vi "4ChNCS_BIOPAC_Zijing_amp_ph.vi"() -> ()   [LabVIEW 2016]
uses:
  <vilib>/measure/NI_MABase.lvlib
  <instrlib>/niUSRP/niUSRP Fetch Rx Data (2D CDB).vi
  <instrlib>/niUSRP/niUSRP Write Tx Data (2D CDB).vi
  <instrlib>/niUSRP/niUSRP Timestamp.ctl
  <instrlib>/niUSRP/niUSRP Configure Time Start Trigger.vi
  <vilib>/Analysis/NI_AALBase.lvlib
  <vilib>/Analysis/3filter.llb/Butterworth Filter (CDB).vi
  <vilib>/Analysis/3filter.llb/Filter Passband Type.ctl
  <vilib>/Analysis/3filter.llb/Butterworth Filter (DBL).vi
  C:/Program Files (x86)/BIOPAC Systems, Inc/BIOPAC Hardware API 2.2 Education/x64/mpdev.dll
  <vilib>/sound2/lvsound2.llb/Sampling Mode.ctl
  <vilib>/sound2/lvsound2.llb/Sound File Info (path).vi
  <vilib>/sound2/lvsound2.llb/Sound File Read Open.vi
  <vilib>/sound2/lvsound2.llb/Sound Output Write (DBL).vi
  <vilib>/sound2/lvsound2.llb/Sound File Read (DBL).vi
  <vilib>/Analysis/NI_AALPro.lvlib
  <vilib>/Platform/browser.llb/Open URL in Default Browser (string).vi
  <vilib>/Utility/miscctls.llb/LVDateTimeRec.ctl
panel:
  out "Wave size/ DS":dbl=10000.0 format="%#_6p"
  out "Tx ch1  ph":cdb[](array[numeric])
  out "Tx ch2  ph":cdb[](array[numeric])
  out "Tx ch4 ph":cdb[](array[numeric])
  out "Tx ch3  ph":cdb[](array[numeric])
  in  "Mute":bool
  out "Play Sound":bool=TRUE
  in  "bottom filter":T1
  in  "top filter":T1=enum."Bandpass"
  out "Acq Started":bool
  out "# BIO View Q":i32
  out "# BIO Buffer":i32
  out "Boolean":bool=TRUE
  out "Disconnecting":bool
  out "Stopping":bool
  out "Connecting":bool
  out "Disconnected":bool
  in  "Show BIO":bool
  out "# BIOViewQ2":i32
  out "Array 1 View":dbl[](graph)
  out "Array 2 View":dbl[](graph)
  out "Array 3 View":dbl[](graph)
  out "Array 4 View":dbl[](graph)
  out "View Array Size":i32
  out "# Elements in Array":i32
  out "ACQ -# Elements":i32
  out "Receive Success":bool
  out "# ACQ cycles":i32
  out "Bytes Read":i32
  out "Bytes To Read":i32
  out "Receive Total Size":dbl format="%#_13g"
  out "Receiving":bool
  in  "Start Acquisition":bool
  in  "Disconnect":bool
  out "ACQ ms":dbl=250.0 format="%#_13g"
  in  "Stop Acquisition":bool
  out "Connected":bool
  in  "Sample Rate":dbl=1.0 caption="ms/sample" min=0.0
  in  "Analog Channels":i32[](array[numeric])=[1, 1, 1, 1]
  out "# Channels":dbl format="%#_13g"
  out "BIO Connect":i32
  in  "BIO Connect":bool=TRUE
  in  "OpenHTML":bool=TRUE
  in  "Abd (cm)":string="0"
  in  "Thorax (cm)":string="0"
  in  "Comments":string
  in  "Weight (lbs)":string="0"
  in  "Age (yrs)":string="0"
  in  "Sex":string(combo)="Female"
  in  "Height (cm)":string="0"
  in  "Case #":string="14"
  out "Start Time":T2
  out "Total Routine Time":dbl(slide) scale=0.0..300.0
  out "Elapsed Time":dbl caption="Elapsed Time (s)"
  out "Next Instruction":string
  out "Current Instruction":string
  in  "Routine Selection":T3(ring)
  out "Current Routine":string
  out "Tx3Rx4":dbl[](graph)
  out "Tx4Rx3":dbl[](graph)
  out "ChAmp":dbl[][](array[numeric])=[[1.7262327066457893e-05, 1.899698926539768e-05, 2.131979680782845e-05, 2.7507513862708948e-05, 3.236234947998919e-05, 3.384280863448985e-05, 3.3113712649913256e-05, 2.8744318806479064e-05, 2.4117959107532184e-05, 2.0714217164135817e-05, 1.7964639969242282e-05, 1.4127881869429752e-05, 1.5692535768228094e-05, 2.4152619914305532e-05, 2.8339686382715385e-05, 2.606906286720416e-05, 2.1755918570529384e-05, 2.0929028564145826e-05, 2.2419410493859248e-05, 2.1786896096171967e-05, 1.7145005999174206e-05, 1.5886785364638103e-05, 1.995380091360238e-05, 1.96084446445408e-05, 1.3881312052638574e-05, 5.368463432831762e-06, 7.886976522489036e-06, 1.718108126568357e-05, 1.984430714817916e-05, 1.8874058751572535e-05, 1.7869312672433515e-05, 1.7356735499504872e-05, 2.065235332503479e-05, 2.1951680154988656e-05, 2.0363547237431346e-05, 2.1229264430323524e-05, 2.188656276617781e-05, 2.1477411495382004e-05, 1.913194947952161e-05, 1.374906879007994e-05, 1.084407557924396e-05, 1.0538448835067238e-05, 1.3462486513328936e-05, 1.979383250422823e-05, 2.381539261154395e-05, 2.2167223174073578e-05, 1.7644503717147575e-05, 1.870536234643517e-05, 2.2751950524913166e-05, 2.340432192813861e-05, 2.2468849270761083e-05, 2.4188550691353842e-05, 2.7519058552290856e-05, 3.1102581077866726e-05, 3.580393911829494e-05, 3.78912649503874e-05, 3.327873597801261e-05, 2.4510981949940783e-05, 1.8465065354817837e-05, 1.7132224969133005e-05, 1.7642310138371268e-05, 1.88142956741822e-05, 1.560032046277488e-05, 9.753217862235494e-06, 1.2015090850038981e-05, 1.776834560720681e-05, 2.4803861691952522e-05, 2.8043624192078222e-05, 2.684382525540612e-05, 2.3530222840588965e-05, 2.0528849124310057e-05, 1.9668374613316667e-05, 1.9146637114645684e-05, 1.5474488036915515e-05, 1.739488550213199e-05, 2.5095299380068926e-05, 3.2858145215540916e-05, 3.439509649081835e-05, 2.6143868318774837e-05, 1.7977385637690134e-05, 1.6384181575586158e-05, 1.4888284293264162e-05, 1.1597491470576354e-05, 1.1445555578759772e-05, 1.4980688444081562e-05, 1.909173519498907e-05, 1.9461150455264684e-05, 1.845876729070065e-05, 1.8005010185132642e-05, 1.9028924898462435e-05, 1.7575955788217445e-05, 1.4184298105937452e-05, 9.414371560237339e-06, 5.4356042784590255e-06, 8.10928562517548e-06, 9.28876849225871e-06, 8.695785214389758e-06, 1.2695777397634576e-05, 1.6809431598631123e-05, 2.1908643727461497e-05], [0.39904903865563796, 0.39903176051530775, 0.39902405260596024, 0.3990221650023599, 0.3990182934858042, 0.39901299641778676, 0.39900459263010085, 0.39899398548309095, 0.3989851312683333, 0.3989817758172843, 0.39898441600096285, 0.3989920701551657, 0.3989957319087615, 0.3989970252526829, 0.3990014639144786, 0.3990082495650084, 0.39901677157837184, 0.39902202434845035, 0.3990170521098724, 0.3990061914814684, 0.39899957115083645, 0.39900163440594105, 0.39901134932465093, 0.3990245430143365, 0.3990299364956871, 0.3990206423396574, 0.39901294696264844, 0.399015237964853, 0.3990195320664335, 0.3990239908891069, 0.39902678858482366, 0.3990303142377581, 0.3990363654196349, 0.39903798034344395, 0.39903568308022536, 0.3990295778239386, 0.3990213145612541, 0.3990115641317417, 0.3990031911721688, 0.3990044335692754, 0.3990142055365442, 0.3990231880559529, 0.3990294810791408, 0.39903152543597487, 0.3990303417237137, 0.39902587131491124, 0.39902317862698444, 0.3990231908517323, 0.3990187535042287, 0.39901147460102687, 0.39900466569609977, 0.399000198693456, 0.398994572076958, 0.39898792975360287, 0.39898351183081265, 0.39898252129559103, 0.3989860199605185, 0.3989908704807006, 0.39899345184972185, 0.39899268675930705, 0.39898929894357515, 0.39898974479144206, 0.3989970434213525, 0.39900457970685, 0.3990084272376425, 0.3990059437407563, 0.39900092658003017, 0.3989998521554356, 0.3989999155043143, 0.39900335732390085, 0.3990086633280822, 0.39901161043288735, 0.3990153435576799, 0.3990232290578827, 0.39902895125044885, 0.3990233171970213, 0.39901091768095076, 0.3989963560226853, 0.3989823146041765, 0.39898013105698543, 0.39899131681473166, 0.3990088743561722, 0.39902163871137375, 0.39902552269435965, 0.3990216751013488, 0.3990108271690995, 0.3989999368161602, 0.39899179748001445, 0.3989869444795569, 0.3989823014007489, 0.3989811018380635, 0.3989866085692465, 0.3989974881575293, 0.399009653455826, 0.39902039237597164, 0.39903113834388676, 0.39903799466445666, 0.39903656085835637, 0.39902912933239515, 0.3990196685727854], [0.5089284260094796, 0.5089413529092005, 0.5089385924023097, 0.5089461735853302, 0.5089333321440155, 0.5089367652503622, 0.5089376331435306, 0.5089306671430541, 0.508949239645895, 0.5089486561361645, 0.5089529378833244, 0.5089419476875585, 0.5089298840108731, 0.5089475772042052, 0.5089441426339854, 0.5089427381450184, 0.5089483329108746, 0.5089280151098653, 0.5089336602793385, 0.5089062019851882, 0.5089074628030626, 0.5088932174425751, 0.5088701289561509, 0.5088760830698362, 0.5088683341509143, 0.5088818393635381, 0.5089000365985035, 0.5088962730652971, 0.5089053012825656, 0.5088919060061875, 0.5088858810710211, 0.5088778714303226, 0.508862396898039, 0.5088799706522465, 0.508890020250467, 0.5089068411749241, 0.508910151200762, 0.5088879724716624, 0.5088963605339264, 0.5088989546591678, 0.5089079531975655, 0.5089307483176185, 0.5089353690581762, 0.5089322510910641, 0.5089226818391756, 0.5089231205950179, 0.5089421889187917, 0.5089302121637822, 0.5089288553338916, 0.5089136387417116, 0.5088923938634197, 0.5088806790242092, 0.5088543127997475, 0.5088388632427274, 0.5088290815518671, 0.5088136498514574, 0.508828716232115, 0.5088373004254244, 0.5088536031198835, 0.5088663652543981, 0.5088663647379902, 0.5088663839922184, 0.5088589552438861, 0.5088642449634635, 0.5088725023266256, 0.5088718014416865, 0.5088674063260687, 0.5088515437004615, 0.5088682831786894, 0.5088713788197812, 0.5088809924897628, 0.508878513506942, 0.5088771181893693, 0.5088848435184512, 0.5088770842370816, 0.5088914766511436, 0.5089003523667647, 0.5089066301516674, 0.5089314320882471, 0.5089402101447223, 0.508962553406896, 0.5089753861787446, 0.5089593307295952, 0.5089478542324088, 0.5089278310589712, 0.5089248500720587, 0.5089163513653545, 0.5089005689237424, 0.5089083211616405, 0.5088993300683022, 0.5088927412237987, 0.5088830866377116, 0.5088718481995638, 0.5088897909905771, 0.5088809733102648, 0.5088790935282286, 0.5088680814653207, 0.5088523600270333, 0.5088613943195607, 0.5088543176402154], [2.0662941946213977e-05, 2.282608405319783e-05, 2.237600508813514e-05, 2.2542693256186783e-05, 2.041826329305299e-05, 1.6288400811782785e-05, 1.0891495139698275e-05, 1.4190599881567273e-05, 1.8742691366266016e-05, 1.8736119036749436e-05, 1.741774537028846e-05, 1.5658954058158222e-05, 1.5904856683822096e-05, 1.6871005066910787e-05, 1.5599249074465836e-05, 1.3520520470394872e-05, 1.3927163947888679e-05, 1.5334805249818678e-05, 1.4564830067379515e-05, 9.817520346860189e-06, 1.3098820613974226e-05, 1.929550220456421e-05, 2.3072255815616586e-05, 2.4321951176986116e-05, 2.3250917563816834e-05, 2.1644284217119052e-05, 1.7041306350033735e-05, 1.0688883027066213e-05, 9.28433634468159e-06, 1.1420718289762068e-05, 1.7056250213804775e-05, 1.9836991189555113e-05, 1.746716828521344e-05, 1.2441527630540996e-05, 8.566795426917848e-06, 9.815076354382859e-06, 1.0229272880058857e-05, 9.936691802926115e-06, 1.536494187514889e-05, 2.3346259934086635e-05, 2.7477587888222747e-05, 2.882421007601368e-05, 2.763067836551142e-05, 2.1577345489474273e-05, 1.3485424327083916e-05, 9.52579824483287e-06, 1.3113651673496717e-05, 1.5276095683726537e-05, 1.6308973250379756e-05, 1.8045078515596545e-05, 1.7849042225306495e-05, 1.2607829522468473e-05, 7.109107971268437e-06, 6.6038815895810515e-06, 6.924972052119899e-06, 4.965235247536195e-06, 5.757305113334596e-06, 9.21497446069365e-06, 9.781248515919794e-06, 1.0683021318304504e-05, 1.196938592791573e-05, 1.159802409297526e-05, 1.012272777630437e-05, 9.65935822948268e-06, 1.4116839432017005e-05, 1.847684147148342e-05, 1.6783927528588872e-05, 1.0863513026975652e-05, 7.650914818223192e-06, 9.456183557358687e-06, 1.0426180609097815e-05, 8.567604650724215e-06, 8.546559610017728e-06, 1.2946532793024891e-05, 1.7245567743458815e-05, 2.0097444147186203e-05, 2.0459407417437442e-05, 1.9957232554286306e-05, 1.996659645997603e-05, 1.7332136966233293e-05, 1.5115608112097958e-05, 1.762095864401886e-05, 1.992020410454883e-05, 2.0585166404108466e-05, 2.212056735942569e-05, 2.2957279986002272e-05, 2.3103396847026532e-05, 2.320807116373638e-05, 2.0818984342366494e-05, 1.789850158592137e-05, 1.64936985167028e-05, 1.4204813599995013e-05, 1.2878752736428332e-05, 1.4757379916553103e-05, 1.713867099725903e-05, 1.6105166890214558e-05, 1.20593443919334e-05, 1.2171370167939264e-05, 1.2336933066341984e-05, 1.1620987924410626e-05]]
  out "Output":bool=TRUE
  out "Ch4 Amplitude":dbl step=0.05 format="%#.6g"
  out "Ch3 Amplitude":dbl=0.25 step=0.05 format="%#.6g"
  out "Ch2 Amplitude":dbl=0.6 step=0.05 format="%#.6g"
  out "Ch1 Amplitude":dbl step=0.05 format="%#.6g"
  out "Tx1Rx2":dbl[](graph)
  out "Tx2Rx1":dbl[](graph)
  out "Dis Sampling Rate":dbl=1000.0 format="%#_6p"
  in  "DownSamplingRatio 2":i32=10
  out "Sampling Rate":dbl=10000.0 format="%#_6p"
  out "Flush":bool
  out "8 Ch Heart":dbl[][](array[numeric])
  out "NCS Save Loops":i32=56132
  out "Save":bool
  out "# NCS Buffer":i32
  out "Buffer":bool
  in  "fl Bottom":dbl=10.0 format="%0.4f"
  in  "fh Bottom":dbl=20.0 format="%0.2f"
  in  "DownSamplingRatio1":i32=200
  in  "fl Top":dbl=4.0 format="%0.4f"
  in  "fh Top":dbl=20.0 format="%0.2f"
  out "# elements in view queue":i32
  out "DownSamplingRatio":i32=100
  out "BW/2":dbl=1000.0
  out "# IQ queue Ch 2":i32
  out "# IQ queue Ch 1":i32
  in  "Dis2":bool=TRUE
  in  "Dis1":bool=TRUE
  out "IQ Graph 2":dbl[][](graph)
  out "IQ Graph":dbl[][](graph)
  out "Tx2 Waveform":cdb[][](array[numeric])
  out "Tx1 Waveform":cdb[][](array[numeric])
  in  "Ch3&4 carrier frequency [Hz] 2":dbl=1000000000.0 format="%#_6p"
  in  "Ch1&2 carrier frequency [Hz]":dbl=900000000.0 format="%#_6p"
  in  "Rx2 Gain 2":dbl=15.0 format="%#_6f"
  in  "Tx2 Gain 2":dbl=20.0 format="%#_6f"
  in  "Rx1 Gain 2":dbl=15.0 format="%#_6f"
  in  "Tx1 Gain 2":dbl=20.0 format="%#_6f"
  out "error out 2":errorcluster
  in  "Start Trigger Time 2":T4={"whole seconds"=1, "fractional seconds"=0.0}
  in  "Channel 4 Tone Amplitude":dbl=0.5 step=0.05 format="%#.6g"
  in  "Channel 4 Tone Frequency":dbl=430000.0 format="%#_6p"
  in  "Channel 3 Tone Amplitude":dbl=0.5 step=0.05 format="%#.6g"
  in  "Channel 3 Tone Frequency":dbl=473000.0 format="%#_6p"
  out "Tx2 Waveform Graph":waveform(dbl)[](graph)=[{"t0"=timestamp(0.45999999999999996 s since 1904-01-01), "dt"=1e-06, "Y"=array[10000 elements]}, {"t0"=timestamp(0.45999999999999996 s since 1904-01-01), "dt"=1e-06, "Y"=array[10000 elements]}, {"t0"=timestamp(0.45999999999999996 s since 1904-01-01), "dt"=1e-06, "Y"=array[10000 elements]}, {"t0"=timestamp(0.45999999999999996 s since 1904-01-01), "dt"=1e-06, "Y"=array[10000 elements]}]
  in  "Waveform Size 2":dbl=10000.0
  in  "Stop 2":bool
  in  "Device Name 2":refnum<k15>="MyB210_2"
  in  "Tx2 Gain 1":dbl=20.0 format="%#_6f"
  in  "Tx IQ Rate 2":dbl=1000000.0 format="%#_6p"
  in  "Rx2 Gain 1":dbl=15.0 format="%#_6f"
  in  "Rx IQ Rate 2":dbl=1000000.0 format="%#_6p"
  out "error out 1":errorcluster
  in  "Start Trigger Time":T4={"whole seconds"=1, "fractional seconds"=0.0}
  in  "Stop":bool
  in  "Channel 2 Tone Amplitude":dbl=0.5 step=0.05 format="%#.6g"
  in  "Channel 2 Tone Frequency":dbl=440000.0 format="%#_6p"
  in  "Channel 1 Tone Amplitude":dbl=0.5 step=0.05 format="%#.6g"
  in  "Channel 1 Tone Frequency":dbl=355000.0 format="%#_6p"
  out "Tx1 Waveform Graph":waveform(dbl)[](graph)=[{"t0"=timestamp(0.45999999999999996 s since 1904-01-01), "dt"=1e-06, "Y"=array[10000 elements]}, {"t0"=timestamp(0.45999999999999996 s since 1904-01-01), "dt"=1e-06, "Y"=array[10000 elements]}, {"t0"=timestamp(0.45999999999999996 s since 1904-01-01), "dt"=1e-06, "Y"=array[10000 elements]}, {"t0"=timestamp(0.45999999999999996 s since 1904-01-01), "dt"=1e-06, "Y"=array[10000 elements]}]
  in  "Waveform Size 1":dbl=10000.0
  in  "Device Name":refnum<k15>="MyB210_1"
  in  "Tx1 Gain 1":dbl=20.0 format="%#_6f"
  in  "Tx IQ Rate 1":dbl=1000000.0 format="%#_6p"
  in  "Rx1 Gain 1":dbl=15.0 format="%#_6f"
  in  "Rx IQ Rate 1":dbl=1000000.0 format="%#_6p"
  # "Misc"
  # "Tx Waveform"
  # "IQ waveform"
  # "NCS"
  # "Channel Settings"
  # "Channel 1"
  # "Device Settings"
  # "BIO"
  # "Channel 2"
  # "Filters"
  # "Buffers"
  # "BIOPAC Connection"
  # "Channel 3"
  # "Post Study Survey:"
  # "https://cornell.qualtrics.com/jfe/form/SV_9QryoqkUKquSXD7"
  # "Channel 4"
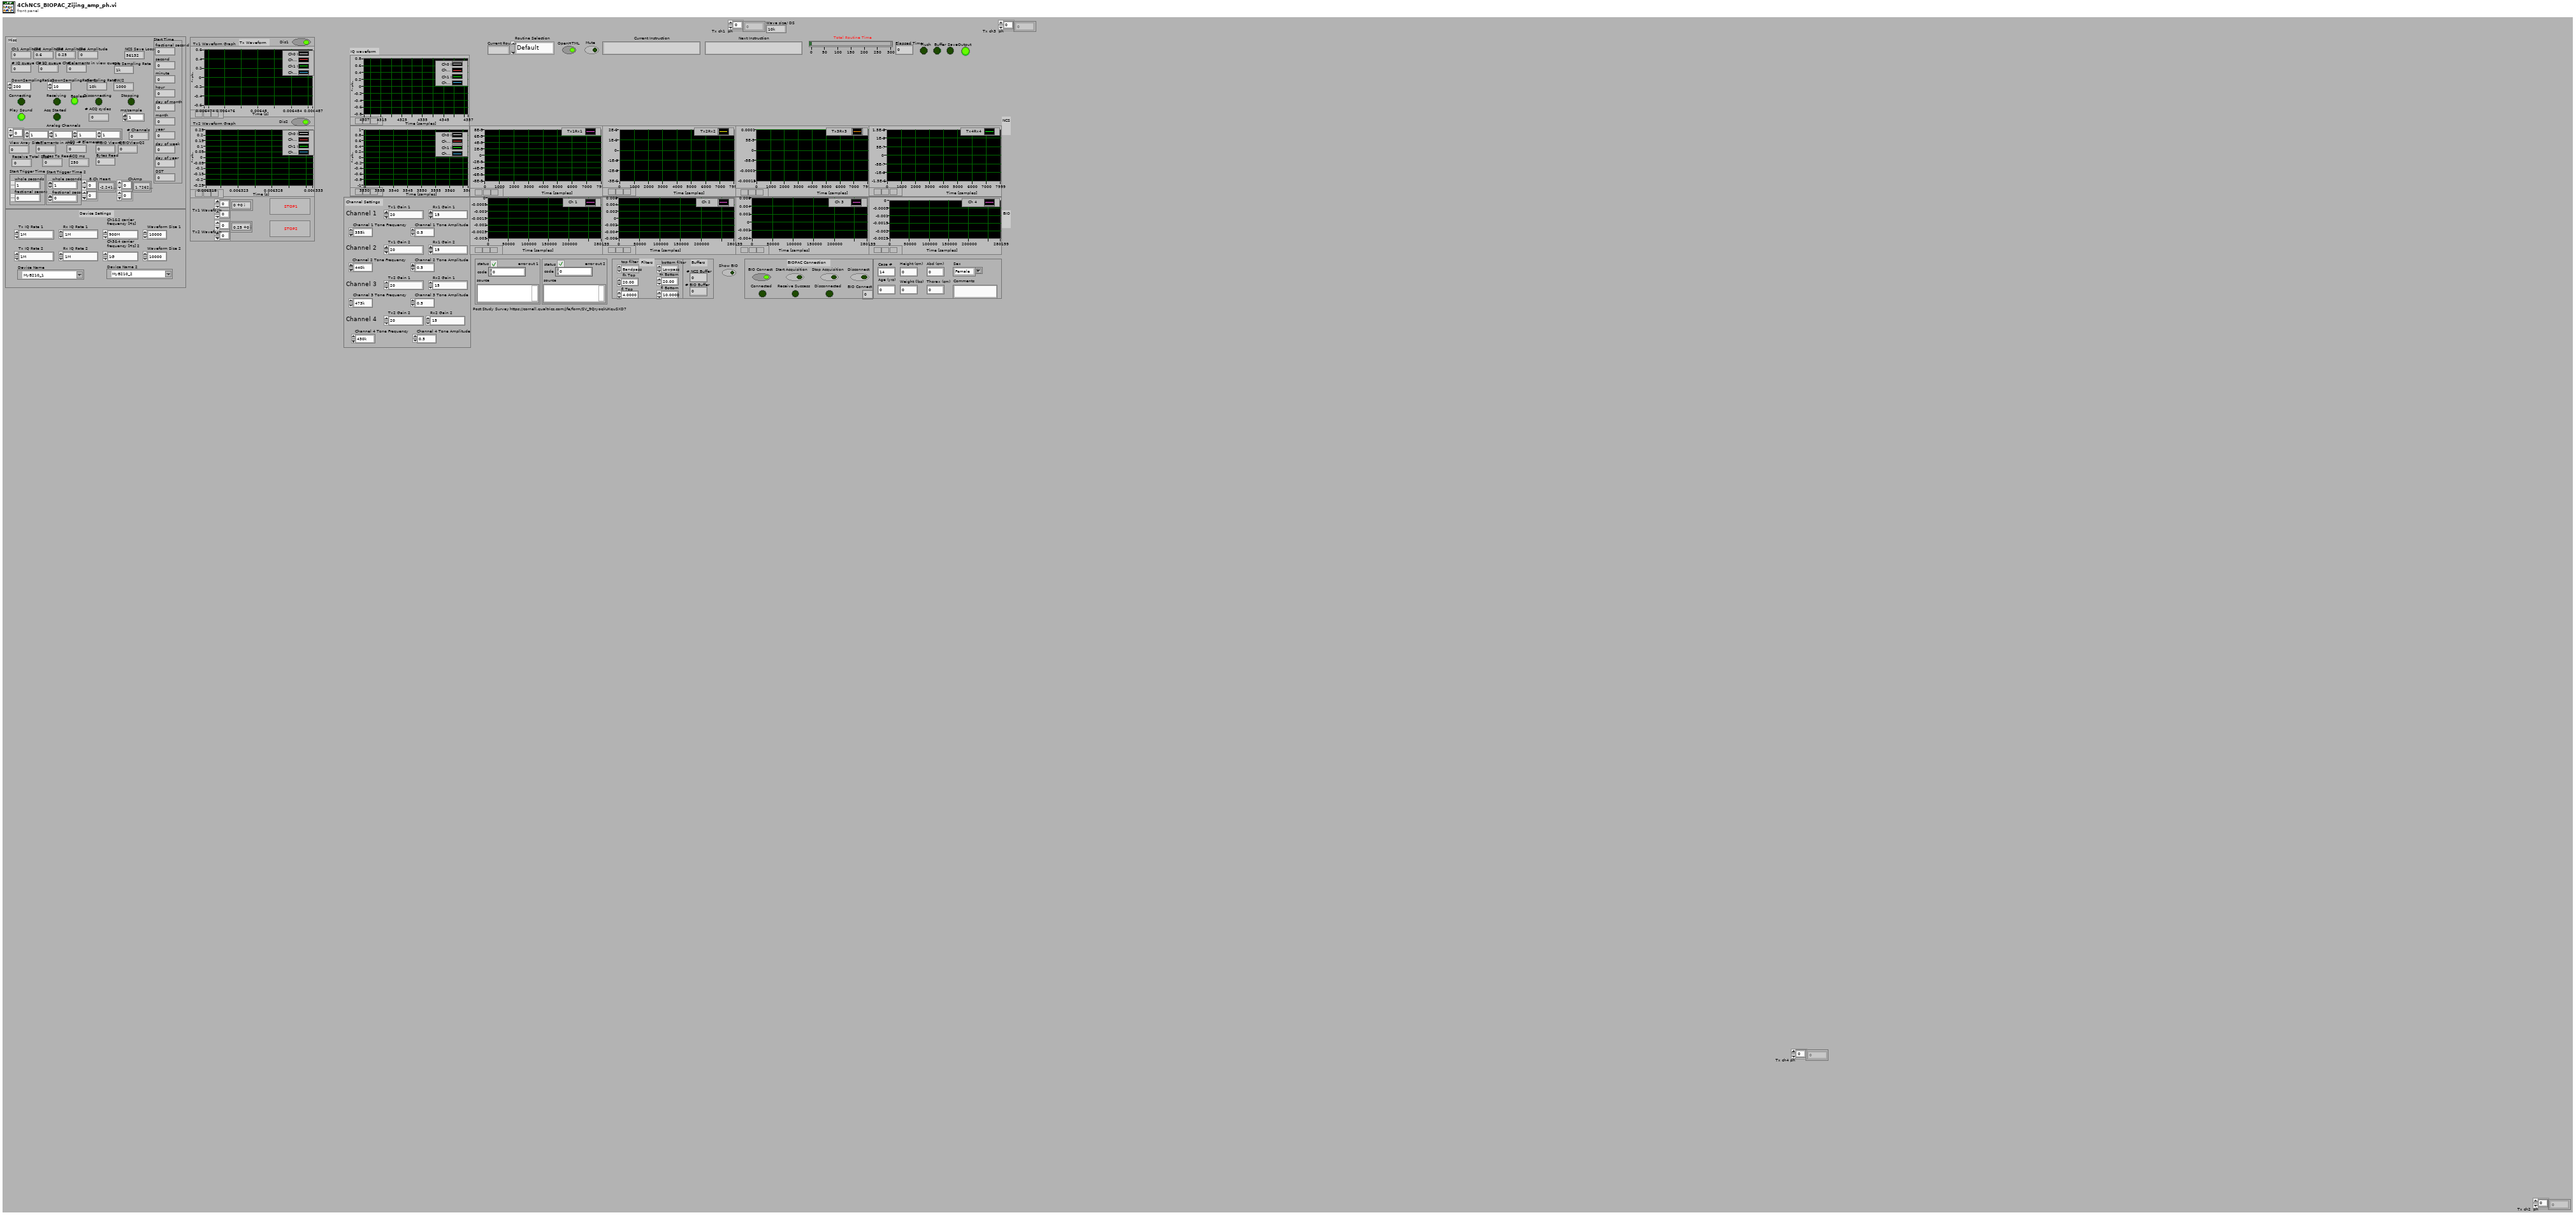
[diagram p1: front panel]
types:
  T1 = typedef "NI_AALBase.lvlib/Filter Passband Type.ctl" = enum32{"Lowpass", "Highpass", "Bandpass", "Bandstop"}
  T2 = typedef "LVDateTimeRec.ctl" = cluster{"fractional second":dbl, "second":i32, "minute":i32, "hour":i32, "day of month":i32, "month":i32, "year":i32, "day of week":i32, "day of year":i32, "DST":i32}
  T3 = enum16{"Default", "Test Run", "Training", "Routine 1", "Routine 2", "Routine 3", "Routine 4", "Routine 5a", "Routine 5b"}
  T4 = typedef "niUSRP Timestamp.ctl" = cluster{"whole seconds":u64, "fractional seconds":dbl}
  T5 = typedef "Sampling Mode.ctl" = i32
  T6 = typedef "Sound Data Format.ctl" = cluster{"sample rate (S/s)":dbl, "number of channels":i32, "bits per sample":i32}
  T7 = typedef "Sound File Refnum.ctl" = refnum<file>
  T8 = typedef "Sound Output Task ID.ctl" = u32
  T9 = enum16{"open", "open or create", "create or replace", "create", "open (read-only)"}
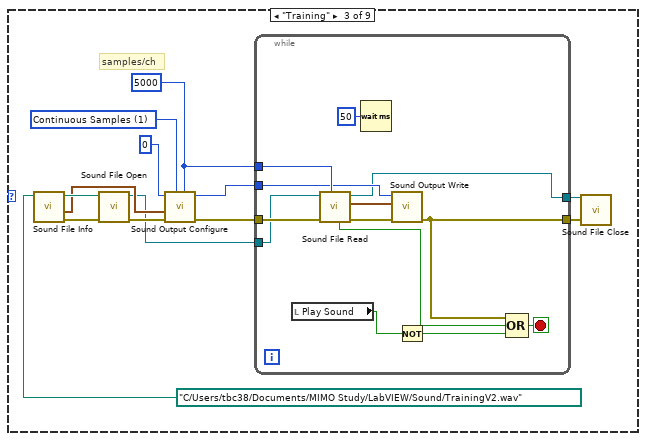
[diagram p4: hidden frame]
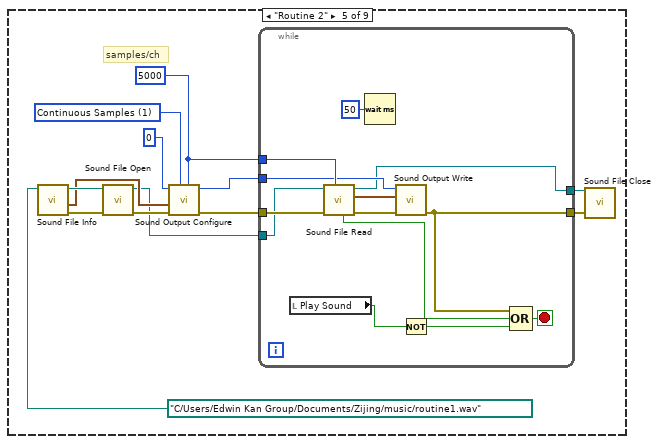
[diagram p6: hidden frame]
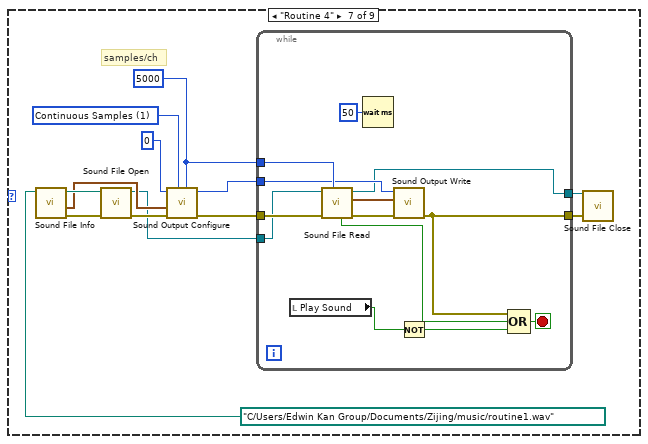
[diagram p8: hidden frame]
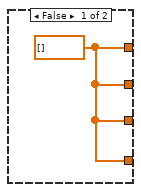
[diagram p11: hidden frame]
diagram:
  w1 = FALSE
  w29 = enum16{"Default"}."Default"
  w26 = 0.0 ("element")
  w27 = 800 ("dimension size")
  w33 = 4 ("dimension size")
  (unwired) 10
  w85 = "RX2"  # Tx active antenna
  w86 = "RX2"  # Tx active antenna
  w142 = 1 items=["Now", "Next Timebase Edge"] ("apply timestamp")
  w114 = "TX1"  # Tx active antenna
  w208 = 1 items=["Now", "Next Timebase Edge"] ("apply timestamp")
  w180 = "TX1"  # Tx active antenna
  # "Sound"
  # "Get it so that it acquires the proper number of cycles for the routine time. Front should be save synchronized"
  # "BIOPAC QUEUE"
  # "Current Sync Method:\nStart Buffering as soon as Acquisition Starts"
  # "Biopac Code. Use the flags to switch between these loops.\nCONNECT- Run to connect to the BIOPAC. Acquisition will not start. 'Connect Success' returns the status of this function.\nSTART ACQUISITION- Run to begin acquiring data from the BIOPAC. SYNCHRONIZATION IS IMPORTANT HERE.\nSTOP ACQUISITION- Run to stop acquiring data. The BIOPAC will disconnect and reconnect to prepare for another acquisition.\nDISCONNECT- Run to disconnect from BIOPAC. This will prohibit connection until the VI is restarted.\nSHOW/VIEWING- Dequeues the elements and displays them."
  # "Routine selection and implementation Loop"
  # "DownSamplingRatio"
  # "Set the attributes \nspecific to channel 1."
  # "Set the attributes \nspecific to channel 0."
  # "Set the attributes \nused by both Rx channels"
  # "Set the attributes \nspecific to Rx channel 1."
  # "Set the attributes \nspecific to Rx channel 0."
  # "Set the attributes \nspecific to channel 1."
  # "Set the attributes \nspecific to channel 0."
  # "Set the attributes \nused by both Rx channels"
  # "Set the attributes \nspecific to Rx channel 1."
  # "Set the attributes \nspecific to Rx channel 0."
  n1 = local write "BIO Connect"(w1) -> ()
  n2 = local write "Start Acquisition"(w1) -> ()
  n3 = local write "Stop Acquisition"(w1) -> ()
  n4 = local write "Disconnect"(w1) -> ()
  n5 = local write "Show BIO"(w1) -> ()
  n6 = local read "Device Name 2"() -> (w150:refnum<k15>)
  n7 = while {
    stop <- FALSE stop-if-true
    n8 = Wait (ms)(milliseconds to wait=50) -> ()  [unwired: 1 out]
    n9 = Not(x="Mute") -> (.not. x?=w224:bool)
    n10 = case shown="True" w224 {
      frame False {
      }
      frame True {
        n11 = local read "Routine Selection"() -> (w227:T3)
        n12 = case shown="\"Default\", Default" w227 {
          frame "Default", Default {
          }
          frame "Test Run" {
          }
          frame "Training" {
            w231 = 5000
            w234 = T5 1 items=["Finite Samples", "Continuous Samples"] ("sample mode")
            # "samples/ch"
            n13 = call-poly <vilib>:"Sound File Info.vi"("path"=path "C:/Users/tbc38/Documents/MIMO Study/LabVIEW/Sound/TrainingV2.wav") -> ("error out"=w239:errorcluster, "sound format"=w235:T6, "path out"=w240:path)  [unwired: 7 in, 1 out]
            n14 = call-poly <vilib>:"Sound File Open.vi"("error in (no error)"=w239, "path"=w240) -> ("error out"=w238:errorcluster, "sound file refnum"=w230:T7)  [unwired: 8 in]
            n15 = call <vilib>:"Sound Output Configure.vi"("number of samples/ch"=w231, "sample mode"=w234, "error in (no error)"=w238, "sound format"=w235, "device ID"=u32 0) -> ("error out"=w233:errorcluster, "task ID"=w232:T8)  [unwired: 5 in]
            n16 = while {
              tunnel: w233 -> [w251]
              tunnel: w232 -> [w252]
              tunnel: w231 -> [w253]
              tunnel: w230 -> [w250]
              tunnel: [w244] -> w229
              tunnel: [w248] -> w228
              stop <- w242 stop-if-true
              n17 = local read "Play Sound"() -> (w241:bool)
              n18 = call-poly <vilib>:"Sound File Read.vi"("number of samples/ch (-1: all)"=w253, "error in (no error)"=w251, "sound file refnum"=w250) -> ("error out"=w247:errorcluster, "data"=w246:waveform(dbl)[], "sound file refnum out"=w248:T7, "end of file?"=w245:bool)  [unwired: 4 in, 1 out]
              n19 = Wait (ms)(milliseconds to wait=50) -> ()  [unwired: 1 out]
              n20 = call-poly <vilib>:"Sound Output Write.vi"("error in (no error)"=w247, "data"=w246, "task ID"=w252) -> ("error out"=w244:errorcluster)  [unwired: 7 in, 1 out]
              n21 = Not(x=w241) -> (.not. x?=w243:bool)
              n22 = Compound Arithmetic op=OR(w244, w245, w243) -> (w242:bool)
            }
            n23 = call <vilib>:"Sound File Close.vi"("error in (no error)"=w229, "sound file refnum"=w228) -> ()  [unwired: 9 in, 1 out]
          }
          frame "Routine 1" {
          }
          frame "Routine 2" {
            w257 = 5000
            w260 = T5 1 items=["Finite Samples", "Continuous Samples"] ("sample mode")
            # "samples/ch"
            n24 = call-poly <vilib>:"Sound File Info.vi"("path"=path "C:/Users/Edwin Kan Group/Documents/Zijing/music/routine1.wav") -> ("error out"=w265:errorcluster, "sound format"=w261:T6, "path out"=w266:path)  [unwired: 7 in, 1 out]
            n25 = call-poly <vilib>:"Sound File Open.vi"("error in (no error)"=w265, "path"=w266) -> ("error out"=w264:errorcluster, "sound file refnum"=w256:T7)  [unwired: 8 in]
            n26 = call <vilib>:"Sound Output Configure.vi"("number of samples/ch"=w257, "sample mode"=w260, "error in (no error)"=w264, "sound format"=w261, "device ID"=u32 0) -> ("error out"=w259:errorcluster, "task ID"=w258:T8)  [unwired: 5 in]
            n27 = while {
              tunnel: w259 -> [w277]
              tunnel: w258 -> [w278]
              tunnel: w257 -> [w279]
              tunnel: w256 -> [w276]
              tunnel: [w270] -> w255
              tunnel: [w274] -> w254
              stop <- w268 stop-if-true
              n28 = local read "Play Sound"() -> (w267:bool)
              n29 = call-poly <vilib>:"Sound File Read.vi"("number of samples/ch (-1: all)"=w279, "error in (no error)"=w277, "sound file refnum"=w276) -> ("error out"=w273:errorcluster, "data"=w272:waveform(dbl)[], "sound file refnum out"=w274:T7, "end of file?"=w271:bool)  [unwired: 4 in, 1 out]
              n30 = Wait (ms)(milliseconds to wait=50) -> ()  [unwired: 1 out]
              n31 = call-poly <vilib>:"Sound Output Write.vi"("error in (no error)"=w273, "data"=w272, "task ID"=w278) -> ("error out"=w270:errorcluster)  [unwired: 7 in, 1 out]
              n32 = Not(x=w267) -> (.not. x?=w269:bool)
              n33 = Compound Arithmetic op=OR(w270, w271, w269) -> (w268:bool)
            }
            n34 = call <vilib>:"Sound File Close.vi"("error in (no error)"=w255, "sound file refnum"=w254) -> ()  [unwired: 9 in, 1 out]
          }
          frame "Routine 3" {
          }
          frame "Routine 4" {
            w283 = 5000
            w286 = T5 1 items=["Finite Samples", "Continuous Samples"] ("sample mode")
            # "samples/ch"
            n35 = call-poly <vilib>:"Sound File Info.vi"("path"=path "C:/Users/Edwin Kan Group/Documents/Zijing/music/routine1.wav") -> ("error out"=w291:errorcluster, "sound format"=w287:T6, "path out"=w292:path)  [unwired: 7 in, 1 out]
            n36 = call-poly <vilib>:"Sound File Open.vi"("error in (no error)"=w291, "path"=w292) -> ("error out"=w290:errorcluster, "sound file refnum"=w282:T7)  [unwired: 8 in]
            n37 = call <vilib>:"Sound Output Configure.vi"("number of samples/ch"=w283, "sample mode"=w286, "error in (no error)"=w290, "sound format"=w287, "device ID"=u32 0) -> ("error out"=w285:errorcluster, "task ID"=w284:T8)  [unwired: 5 in]
            n38 = while {
              tunnel: w285 -> [w303]
              tunnel: w284 -> [w304]
              tunnel: w283 -> [w305]
              tunnel: w282 -> [w302]
              tunnel: [w296] -> w281
              tunnel: [w300] -> w280
              stop <- w294 stop-if-true
              n39 = local read "Play Sound"() -> (w293:bool)
              n40 = call-poly <vilib>:"Sound File Read.vi"("number of samples/ch (-1: all)"=w305, "error in (no error)"=w303, "sound file refnum"=w302) -> ("error out"=w299:errorcluster, "data"=w298:waveform(dbl)[], "sound file refnum out"=w300:T7, "end of file?"=w297:bool)  [unwired: 4 in, 1 out]
              n41 = Wait (ms)(milliseconds to wait=50) -> ()  [unwired: 1 out]
              n42 = call-poly <vilib>:"Sound Output Write.vi"("error in (no error)"=w299, "data"=w298, "task ID"=w304) -> ("error out"=w296:errorcluster)  [unwired: 7 in, 1 out]
              n43 = Not(x=w293) -> (.not. x?=w295:bool)
              n44 = Compound Arithmetic op=OR(w296, w297, w295) -> (w294:bool)
            }
            n45 = call <vilib>:"Sound File Close.vi"("error in (no error)"=w281, "sound file refnum"=w280) -> ()  [unwired: 9 in, 1 out]
          }
          frame "Routine 5a" {
          }
          frame "Routine 5b" {
          }
        }
      }
    }
  }
  n46 = while {
    stop <- FALSE stop-if-true
    # "STOP ACQUISITION"
    n47 = local read "Connected"() -> (w310:bool)
    n48 = local read "Receiving"() -> (w309:bool)
    n49 = local read "Stopping"() -> (w307:bool)
    n50 = Wait (ms)(milliseconds to wait=100) -> ()  [unwired: 1 out]
    n51 = Not(x=w307) -> (.not. x?=w306:bool)
    n52 = And(x=w309, y=w306) -> (x .and. y?=w308:bool)
    n53 = And(x=w310, y=w308) -> (x .and. y?=w311:bool)
    n54 = And(x="Stop Acquisition", y=w311) -> (x .and. y?=w314:bool)
    n55 = case shown="True" w314 {
      frame False {
      }
      frame True {
        n56 = flat-sequence {
          frame #0 {
            n57 = local write "Stopping"(TRUE) -> ()
            n58 = dll-call lib="C:/Program Files (x86)/BIOPAC Systems, Inc/BIOPAC Hardware API 2.2 Education/x64/mpdev.dll" fn="stopAcquisition" label="stop"() -> ()  [unwired: 4 in, 2 out]
            n59 = local write "Receiving"(FALSE) -> ()
          }
          frame #1 {
            n60 = dll-call lib="C:/Program Files (x86)/BIOPAC Systems, Inc/BIOPAC Hardware API 2.2 Education/x64/mpdev.dll" fn="disconnectMPDev" label="disconnect"() -> ()  [unwired: 4 in, 2 out]
          }
          frame #2 {
            n61 = local read "ACQ ms"() -> (w319:dbl)
            n62 = Add(x=w319, y=200) -> (x+y=w320:dbl)
            n63 = Wait (ms)(milliseconds to wait=w320) -> ()  [unwired: 1 out]
          }
          frame #3 {
            w321 = FALSE
            n64 = local write "Stop Acquisition"(w321) -> ()
            n65 = local write "Stopping"(w321) -> ()
            n66 = local write "Connected"(w321) -> ()
            n67 = local write "Receive Success"(w321) -> ()
          }
        }
      }
    }
  }
  n68 = while {
    stop <- FALSE stop-if-true
    # "CONNECT"
    n69 = local read "Connecting"() -> (w330:bool)
    n70 = local read "Connected"() -> (w329:bool)
    n71 = local read "Disconnected"() -> (w326:bool)
    n72 = Wait (ms)(milliseconds to wait=500) -> ()  [unwired: 1 out]
    n73 = Not(x=w330) -> (.not. x?=w328:bool)
    n74 = Not(x=w329) -> (.not. x?=w325:bool)
    n75 = Not(x=w326) -> (.not. x?=w324:bool)
    n76 = And(x=w325, y=w324) -> (x .and. y?=w323:bool)
    n77 = And(x=w328, y=w323) -> (x .and. y?=w327:bool)
    n78 = And(x="BIO Connect", y=w327) -> (x .and. y?=w331:bool)
    n79 = case shown="True" w331 {
      frame False {
      }
      frame True {
        n80 = flat-sequence {
          frame #0 {
            n81 = local write "BIO Connect"(FALSE) -> ()
            n82 = local write "Connecting"(TRUE) -> ()
          }
          frame #1 {
            w341 = u32 1  # MPSUCCESS
            w350 = 10  # Enumeration Value For USB
            w349 = 103  # Enumeration Value for MP36
            n83 = String To Byte Array(string="") -> (unsigned byte array=w347:u8[])
            n84 = dll-call lib="C:/Program Files (x86)/BIOPAC Systems, Inc/BIOPAC Hardware API 2.2 Education/x64/mpdev.dll" fn="connectMPDev" label="connect"("mptype"=w349, "mpcomtype"=w350, "sn"=w347) -> ("return type"=w346:u32)  [unwired: 6 in, 2 out]
            "BIO Connect" <- w346
            n85 = Not Equal?(x=w346, y=w341) -> (x != y?=w345:bool)
            n86 = case shown="True" w345 {
              frame False {
              }
              frame True {
                n87 = flat-sequence {
                  frame #0 {
                    n88 = dll-call lib="C:/Program Files (x86)/BIOPAC Systems, Inc/BIOPAC Hardware API 2.2 Education/x64/mpdev.dll" fn="stopAcquisition" label="stop"() -> ()  [unwired: 4 in, 2 out]
                  }
                  frame #1 {
                    n89 = dll-call lib="C:/Program Files (x86)/BIOPAC Systems, Inc/BIOPAC Hardware API 2.2 Education/x64/mpdev.dll" fn="disconnectMPDev" label="disconnect"() -> ()  [unwired: 4 in, 2 out]
                  }
                }
              }
            }
            n90 = Not(x=w345) -> (.not. x?=w344:bool)
            n91 = case shown="True" w344 {
              tunnel: [w351 w353] -> w342
              tunnel: [w351 w352] -> w343
              frame False {
                w351 = 0
              }
              frame True {
                n92 = flat-sequence {
                  tunnel: [w357] -> w353
                  tunnel: [w359] -> w352
                  frame #0 {
                    n93 = To Double Precision Float(number="Analog Channels") -> (double precision float=w355:dbl[])
                    n94 = Add Array Elements(numeric array=w355) -> (sum=→"# Channels":dbl)
                    n95 = dll-call lib="C:/Program Files (x86)/BIOPAC Systems, Inc/BIOPAC Hardware API 2.2 Education/x64/mpdev.dll" fn="setAcqChannels" label="set analog CH"("aCH"="Analog Channels") -> ("return type"=w357:u32)  [unwired: 4 in, 2 out]
                  }
                  frame #1 {
                    n96 = dll-call lib="C:/Program Files (x86)/BIOPAC Systems, Inc/BIOPAC Hardware API 2.2 Education/x64/mpdev.dll" fn="setSampleRate" label="set sample rate"("rate"="Sample Rate") -> ("return type"=w359:u32)  [unwired: 4 in, 2 out]
                  }
                }
              }
            }
            n97 = Not Equal?(x=w343, y=w341) -> (x != y?=w338:bool)
            n98 = Not Equal?(x=w342, y=w341) -> (x != y?=w337:bool)
            n99 = Not(x=w337) -> (.not. x?=w339:bool)
            n100 = case shown="True" w337 {
              frame False {
              }
              frame True {
                n101 = flat-sequence {
                  frame #0 {
                    n102 = dll-call lib="C:/Program Files (x86)/BIOPAC Systems, Inc/BIOPAC Hardware API 2.2 Education/x64/mpdev.dll" fn="stopAcquisition" label="stop"() -> ()  [unwired: 4 in, 2 out]
                  }
                  frame #1 {
                    n103 = dll-call lib="C:/Program Files (x86)/BIOPAC Systems, Inc/BIOPAC Hardware API 2.2 Education/x64/mpdev.dll" fn="disconnectMPDev" label="disconnect"() -> ()  [unwired: 4 in, 2 out]
                  }
                }
              }
            }
            n104 = case shown="True" w338 {
              frame False {
              }
              frame True {
                n105 = flat-sequence {
                  frame #0 {
                    n106 = dll-call lib="C:/Program Files (x86)/BIOPAC Systems, Inc/BIOPAC Hardware API 2.2 Education/x64/mpdev.dll" fn="stopAcquisition" label="stop"() -> ()  [unwired: 4 in, 2 out]
                  }
                  frame #1 {
                    n107 = dll-call lib="C:/Program Files (x86)/BIOPAC Systems, Inc/BIOPAC Hardware API 2.2 Education/x64/mpdev.dll" fn="disconnectMPDev" label="disconnect"() -> ()  [unwired: 4 in, 2 out]
                  }
                }
              }
            }
            n108 = Not(x=w338) -> (.not. x?=w340:bool)
            n109 = And(x=w340, y=w339) -> (x .and. y?=w336:bool)
            n110 = local write "Connected"(w336) -> ()
          }
          frame #2 {
            n111 = local write "Connecting"(FALSE) -> ()
          }
        }
      }
    }
  }
  n112 = local read "Device Name"() -> (w216:refnum<k15>)
  n113 = call <instrlib>:"niUSRP Open Rx Session.vi"("device names"="Device Name 2") -> ("session handle out"=w141:refnum<k15>, "error out"=w140:errorcluster)  [unwired: 13 in]
  n114 = property class="niUSRP"(reference=w141, error in=w140, "Enabled Channels"="0,1" ("Configuration:Enabled Channels")) -> (reference out=w139:refnum<k15>, error out=w138:errorcluster)
  n115 = call <instrlib>:"niUSRP Open Rx Session.vi"("device names"="Device Name") -> ("session handle out"=w207:refnum<k15>, "error out"=w206:errorcluster)  [unwired: 13 in]
  n116 = property class="niUSRP"(reference=w207, error in=w206, "Enabled Channels"="0,1" ("Configuration:Enabled Channels")) -> (reference out=w205:refnum<k15>, error out=w204:errorcluster)
  n117 = call-poly <instrlib>:"niUSRP Configure Trigger.vi"("session handle"=w139, "start trigger time"="Start Trigger Time 2", "error in (no error)"=w138) -> ("session handle out"=w135:refnum<k15>, "error out"=w134:errorcluster)  [unwired: 11 in]
  n118 = call-poly <instrlib>:"niUSRP Configure Trigger.vi"("session handle"=w205, "start trigger time"="Start Trigger Time", "error in (no error)"=w204) -> ("session handle out"=w201:refnum<k15>, "error out"=w200:errorcluster)  [unwired: 11 in]
  n119 = property class="niUSRP"(reference=w135, error in=w134, "IQ Rate"="Rx IQ Rate 2") -> (reference out=w131:refnum<k15>, error out=w132:errorcluster)
  n120 = property class="niUSRP"(reference=w201, error in=w200, "IQ Rate"="Rx IQ Rate 1") -> (reference out=w197:refnum<k15>, error out=w198:errorcluster)
  n121 = property class="niUSRP" props=["Model", "Reference Frequency Source", "Timebase Clock Source"](reference=w197, error in=w198, "Reference Frequency Source"="RefIn" ("Clocking and Synchronization:Reference Frequency Source"), "Timebase Clock Source"="PpsIn" ("Clocking and Synchronization:Timebase Clock Source")) -> (reference out=w193:refnum<k15>, error out=w194:errorcluster)  [unwired: 1 out]
  n122 = property class="niUSRP" props=["Model", "Reference Frequency Source", "Timebase Clock Source"](reference=w131, error in=w132, "Reference Frequency Source"="RefIn" ("Clocking and Synchronization:Reference Frequency Source"), "Timebase Clock Source"="PpsIn" ("Clocking and Synchronization:Timebase Clock Source")) -> (reference out=w127:refnum<k15>, error out=w128:errorcluster)  [unwired: 1 out]
  n123 = local write "Routine Selection"(w29) -> ()
  n124 = local read "# Channels"() -> (w4:dbl)
  n125 = local read "ACQ ms"() -> (w3:dbl)
  n126 = while {
    shift-right: ["Routine Selection"] -> _
    shift-left: w29 -> [w367]
    stop <- FALSE stop-if-true
    n127 = case shown="\"Routine 5a\"" w367 {
      tunnel: ["Default" w397 "Isovolumetric Training" "Routine1" "Routine2" "Routine3" "Routine4" "Routine5a" "Routine5b"] -> w368
      tunnel: [w383 w397 w406 "normal breathing+speaking" "normal breathing+eating" " exercise" "exercise " "normal breathing+straw" "end"] -> w365
      tunnel: [w370 _ w404 w452 w474 w507 w525 w551 w569] -> w363
      tunnel: [w370 _ w404 w452 w474 w507 w525 w551 w569] -> w364
      tunnel: [w383 w397 w405 " normal breathing" "normal breathing+ speaking" "post-exercise normal breathing" "post exercise -breathing protocol" "normal breathing+mask" "normal breathing with straw"] -> w362
      tunnel: [w382 w396 w403 w450 w479 w505 w530 w554 w573] -> w361
      frame "Default" {
        w370 = 0.0
        w383 = "No instruction"
        # "BIO should not be acquiring"
        # "If BIO is not connected, attempt to reconnect"
        n128 = Seconds To Date/Time(time stamp (now)=0.0) -> (date time rec=w382:T2)  [unwired: 1 in]
        n129 = local read "# NCS Buffer"() -> (w372:i32)
        n130 = Not Equal?(x=w372, y=0) -> (x != y?=w373:bool)
        n131 = local write "BIO Connect"(TRUE) -> ()
        n132 = case shown="True" w373 {
          frame False {
            n133 = local write "Flush"(FALSE) -> ()
          }
          frame True {
            "Flush" <- TRUE
          }
        }
        n134 = local write "Start Acquisition"(FALSE) -> ()
        n135 = local write "Stop Acquisition"(TRUE) -> ()
        "Save" <- FALSE
        "Buffer" <- FALSE
        "Output" <- FALSE
        "Play Sound" <- FALSE
      }
      frame "Test Run" {
        w397 = "Testing"
        # "Start BIO Acquisition"
        n136 = Seconds To Date/Time(time stamp (now)=0.0) -> (date time rec=w396:T2)  [unwired: 1 in]
        n137 = local write "Start Acquisition"(TRUE) -> ()
        n138 = local write "Stop Acquisition"(FALSE) -> ()
        n139 = local write "Play Sound"(FALSE) -> ()
        n140 = local write "Save"(FALSE) -> ()
        n141 = local write "Output"(TRUE) -> ()
        n142 = local write "Flush"(FALSE) -> ()
        n143 = local write "BIO Connect"(FALSE) -> ()
        n144 = local write "Buffer"(FALSE) -> ()
      }
      frame "Training" {
        w401 = 90.0  # Routine Time
        n145 = local read "Output"() -> (w398:bool)
        n146 = Not(x=w398) -> (.not. x?=w399:bool)
        n147 = call "Elapsed Time3"("Time Target (s)"=w401, "Reset"=w399) -> ("Get Start Time (s)"=w402:dbl, "Elapsed Time (s)"=w404:dbl, "Time has Elapsed"=w400:bool)  [unwired: 10 in, 5 out]
        n148 = script code="t = [300, ...\n       310, 313, 316, 319, 322, ...\n       340, 343, 346, 349, 352, ...\n       370, 373, 376, 379, 382, 390]; % 4) Isovol\nt = t-300;\n\nevent =  [0, ...\n                6, 3, 4, 5, 0, ... % 4) Isovol\n                7, 3, 4, 5, 0, ...\n                8, 3, 4, 5, 0, 0]; \n\nfor i = 2:length(t)\n    if ((x>=t(i-1)) &&  (x<t(i)))\n        y = event(i-1);\n        yNext = event(i);\n        % dt = t(i) - t(i-1);\n        break;\n    end\nend" "Routine timing"("x"=w404) -> ("yNext"=w407:dbl, "y"=w408:dbl)  [unwired: 1 in, 1 out]
        n149 = property on="Total Routine Time" class="Slide (strict)"("Scale.Maximum"=w401) -> ()  [unwired: 2 in, 2 out]
        n150 = Seconds To Date/Time(time stamp (now)=w402) -> (date time rec=w403:T2)  [unwired: 1 in]
        n151 = case shown="False" w400 {
          frame False {
            n152 = local write "Play Sound"(TRUE) -> ()
            n153 = local write "Output"(TRUE) -> ()
            n154 = local write "Flush"(FALSE) -> ()
            n155 = local write "Save"(FALSE) -> ()
            n156 = local write "Buffer"(FALSE) -> ()
            n157 = local write "Start Acquisition"(TRUE) -> ()
            n158 = local write "Stop Acquisition"(FALSE) -> ()
            n159 = local write "BIO Connect"(FALSE) -> ()
          }
          frame True {
            n160 = local write "Play Sound"(FALSE) -> ()
            n161 = local write "Buffer"(FALSE) -> ()
            n162 = local write "Output"(FALSE) -> ()
            n163 = local write "Save"(FALSE) -> ()
            n164 = local write "Flush"(FALSE) -> ()
            n165 = local write "Start Acquisition"(FALSE) -> ()
            n166 = local write "Stop Acquisition"(TRUE) -> ()
            n167 = local write "BIO Connect"(FALSE) -> ()
            n168 = local write "Routine Selection"(enum16{"Default"}."Default") -> ()
          }
        }
        n169 = case "Next Instruction" shown="3" w407 {
          tunnel: ["Perform Normal Breathing" "Max Inhale Breath Hold" "Max Exhalation Breath Hold" "Plug Nose. Move air to chest" "Allow abdomen to relax." "Move air to abdomen." "Exhale Fully" "Inhale Fully" "Inhale Partially"] -> w406
          frame 0, Default {
          }
          frame 1 {
          }
          frame 2 {
          }
          frame 3 {
          }
          frame 4 {
          }
          frame 5 {
          }
          frame 6 {
          }
          frame 7 {
          }
          frame 8 {
          }
        }
        n170 = case "Current Instruction" shown="5" w408 {
          tunnel: ["Perform Normal Breathing" "Max Inhale Breath Hold" "Max Exhalation Breath Hold" "Plug Nose. Move air to chest" "Allow abdomen to relax." "Move air to abdomen." "Exhale Fully" "Inhale Fully" "Inhale Partially"] -> w405
          frame 0, Default {
          }
          frame 1 {
          }
          frame 2 {
          }
          frame 3 {
          }
          frame 4 {
          }
          frame 5 {
          }
          frame 6 {
          }
          frame 7 {
          }
          frame 8 {
          }
        }
      }
      frame "Routine 1" {
        w453 = 300.0  # Routine Time
        # "300"
        # "Supine Breath Monitoring"
        n171 = local read "Output"() -> (w447:bool)
        n172 = Not(x=w447) -> (.not. x?=w448:bool)
        n173 = call "Elapsed Time"("Time Target (s)"=w453, "Reset"=w448) -> ("Get Start Time (s)"=w451:dbl, "Elapsed Time (s)"=w452:dbl, "Time has Elapsed"=w449:bool)  [unwired: 10 in, 5 out]
        n174 = property on="Total Routine Time" class="Slide (strict)"("Scale.Maximum"=w453) -> ()  [unwired: 2 in, 2 out]
        n175 = Seconds To Date/Time(time stamp (now)=w451) -> (date time rec=w450:T2)  [unwired: 1 in]
        n176 = case shown="True" w449 {
          frame False {
            # "Routine Not Done. Continue buffering."
            n177 = flat-sequence {
              frame #0 {
                n178 = local write "Start Acquisition"(TRUE) -> ()
                n179 = local write "Stop Acquisition"(FALSE) -> ()
                n180 = local write "Output"(TRUE) -> ()
                n181 = local write "BIO Connect"(FALSE) -> ()
                n182 = local write "Play Sound"(TRUE) -> ()
              }
              frame #1 {
                n183 = local write "Buffer"(TRUE) -> ()
              }
            }
          }
          frame True {
            # "Routine done. Save."
            n184 = flat-sequence {
              frame #0 {
                n185 = local write "Buffer"(FALSE) -> ()
              }
              frame #1 {
                n186 = local write "Start Acquisition"(FALSE) -> ()
                n187 = local write "Stop Acquisition"(TRUE) -> ()
                n188 = local write "Output"(FALSE) -> ()
              }
              frame #2 {
                n189 = local write "Save"(TRUE) -> ()
              }
              frame #3 {
                n190 = Wait (ms)(milliseconds to wait=500) -> ()  [unwired: 1 out]
              }
              frame #4 {
                n191 = local write "Flush"(TRUE) -> ()
              }
              frame #5 {
                n192 = local write "Flush"(FALSE) -> ()
                n193 = local write "Save"(FALSE) -> ()
              }
              frame #6 {
                n194 = local write "Routine Selection"(enum16{"Default"}."Default") -> ()
                n195 = local write "Play Sound"(FALSE) -> ()
              }
            }
          }
        }
      }
      frame "Routine 2" {
        w480 = 180.0  # Routine Time
        # "Seated Breath Monitoring"
        n196 = local read "Output"() -> (w476:bool)
        n197 = Not(x=w476) -> (.not. x?=w475:bool)
        n198 = call "Elapsed Time2"("Time Target (s)"=w480, "Reset"=w475) -> ("Get Start Time (s)"=w478:dbl, "Elapsed Time (s)"=w474:dbl, "Time has Elapsed"=w477:bool)  [unwired: 10 in, 5 out]
        n199 = property on="Total Routine Time" class="Slide (strict)"("Scale.Maximum"=w480) -> ()  [unwired: 2 in, 2 out]
        n200 = Seconds To Date/Time(time stamp (now)=w478) -> (date time rec=w479:T2)  [unwired: 1 in]
        n201 = case shown="True" w477 {
          frame False {
            # "Routine Not Done. Continue buffering."
            n202 = flat-sequence {
              frame #0 {
                n203 = local write "Play Sound"(TRUE) -> ()
                n204 = local write "Start Acquisition"(TRUE) -> ()
                n205 = local write "Output"(TRUE) -> ()
                n206 = local write "Stop Acquisition"(FALSE) -> ()
                n207 = local write "BIO Connect"(FALSE) -> ()
              }
              frame #1 {
                n208 = local write "Buffer"(TRUE) -> ()
              }
            }
          }
          frame True {
            # "Routine done. Save."
            n209 = flat-sequence {
              frame #0 {
                n210 = local write "Buffer"(FALSE) -> ()
              }
              frame #1 {
                n211 = local write "Output"(FALSE) -> ()
                n212 = local write "Start Acquisition"(FALSE) -> ()
                n213 = local write "Stop Acquisition"(TRUE) -> ()
              }
              frame #2 {
                n214 = local write "Save"(TRUE) -> ()
              }
              frame #3 {
                n215 = Wait (ms)(milliseconds to wait=500) -> ()  [unwired: 1 out]
              }
              frame #4 {
                n216 = local write "Flush"(TRUE) -> ()
              }
              frame #5 {
                n217 = local write "Flush"(FALSE) -> ()
                n218 = local write "Save"(FALSE) -> ()
              }
              frame #6 {
                n219 = local write "Routine Selection"(enum16{"Default"}."Default") -> ()
                n220 = local write "Play Sound"(FALSE) -> ()
              }
            }
          }
        }
      }
      frame "Routine 3" {
        w506 = 300.0  # Routine Time
        # "Supine Heart Monitoring"
        # "180"
        n221 = local read "Output"() -> (w501:bool)
        n222 = Not(x=w501) -> (.not. x?=w502:bool)
        n223 = call "Elapsed Time4"("Time Target (s)"=w506, "Reset"=w502) -> ("Get Start Time (s)"=w504:dbl, "Elapsed Time (s)"=w507:dbl, "Time has Elapsed"=w503:bool)  [unwired: 10 in, 5 out]
        n224 = property on="Total Routine Time" class="Slide (strict)"("Scale.Maximum"=w506) -> ()  [unwired: 2 in, 2 out]
        n225 = Seconds To Date/Time(time stamp (now)=w504) -> (date time rec=w505:T2)  [unwired: 1 in]
        n226 = case shown="True" w503 {
          frame False {
            # "Routine Not Done. Continue buffering."
            n227 = flat-sequence {
              frame #0 {
                w510 = FALSE
                w509 = TRUE
                n228 = local write "Stop Acquisition"(w510) -> ()
                n229 = local write "BIO Connect"(w510) -> ()
                n230 = local write "Play Sound"(w509) -> ()
                n231 = local write "Output"(w509) -> ()
                n232 = local write "Start Acquisition"(w509) -> ()
              }
              frame #1 {
                n233 = local write "Buffer"(TRUE) -> ()
              }
            }
          }
          frame True {
            # "Routine done. Save."
            n234 = flat-sequence {
              frame #0 {
                n235 = local write "Buffer"(FALSE) -> ()
              }
              frame #1 {
                n236 = local write "Play Sound"(FALSE) -> ()
                n237 = local write "Output"(FALSE) -> ()
                n238 = local write "Start Acquisition"(FALSE) -> ()
                n239 = local write "Stop Acquisition"(TRUE) -> ()
              }
              frame #2 {
                n240 = local write "Save"(TRUE) -> ()
              }
              frame #3 {
                n241 = Wait (ms)(milliseconds to wait=500) -> ()  [unwired: 1 out]
              }
              frame #4 {
                n242 = local write "Flush"(TRUE) -> ()
              }
              frame #5 {
                n243 = local write "Flush"(FALSE) -> ()
                n244 = local write "Save"(FALSE) -> ()
              }
              frame #6 {
                n245 = local write "Routine Selection"(enum16{"Default"}."Default") -> ()
              }
            }
          }
        }
      }
      frame "Routine 4" {
        w531 = 180.0  # Routine Time
        # "Seated Heart Monitoring"
        # "300"
        n246 = local read "Output"() -> (w526:bool)
        n247 = Not(x=w526) -> (.not. x?=w527:bool)
        n248 = call "Elapsed Time5"("Time Target (s)"=w531, "Reset"=w527) -> ("Get Start Time (s)"=w529:dbl, "Elapsed Time (s)"=w525:dbl, "Time has Elapsed"=w528:bool)  [unwired: 10 in, 5 out]
        n249 = property on="Total Routine Time" class="Slide (strict)"("Scale.Maximum"=w531) -> ()  [unwired: 2 in, 2 out]
        n250 = Seconds To Date/Time(time stamp (now)=w529) -> (date time rec=w530:T2)  [unwired: 1 in]
        n251 = case shown="False" w528 {
          frame False {
            # "Routine Not Done. Continue buffering."
            n252 = flat-sequence {
              frame #0 {
                w534 = FALSE
                w533 = TRUE
                n253 = local write "Play Sound"(w533) -> ()
                n254 = local write "Stop Acquisition"(w534) -> ()
                n255 = local write "Output"(w533) -> ()
                n256 = local write "Start Acquisition"(w533) -> ()
                n257 = local write "BIO Connect"(w534) -> ()
              }
              frame #1 {
                n258 = local write "Buffer"(TRUE) -> ()
              }
            }
          }
          frame True {
            # "Routine done. Save."
            n259 = flat-sequence {
              frame #0 {
                n260 = local write "Buffer"(FALSE) -> ()
              }
              frame #1 {
                w537 = FALSE
                n261 = local write "Play Sound"(w537) -> ()
                n262 = local write "Output"(w537) -> ()
                n263 = local write "Start Acquisition"(w537) -> ()
                n264 = local write "Stop Acquisition"(TRUE) -> ()
              }
              frame #2 {
                n265 = local write "Save"(TRUE) -> ()
              }
              frame #3 {
                n266 = Wait (ms)(milliseconds to wait=500) -> ()  [unwired: 1 out]
              }
              frame #4 {
                n267 = local write "Flush"(TRUE) -> ()
              }
              frame #5 {
                n268 = local write "Flush"(FALSE) -> ()
                n269 = local write "Save"(FALSE) -> ()
              }
              frame #6 {
                n270 = local write "Routine Selection"(enum16{"Default"}."Default") -> ()
              }
            }
          }
        }
      }
      frame "Routine 5a" {
        w550 = 300.0  # Routine Time
        # "Relaxation"
        # "180"
        n271 = local read "Output"() -> (w547:bool)
        n272 = Not(x=w547) -> (.not. x?=w548:bool)
        n273 = call "Elapsed Time7"("Time Target (s)"=w550, "Reset"=w548) -> ("Get Start Time (s)"=w552:dbl, "Elapsed Time (s)"=w551:dbl, "Time has Elapsed"=w549:bool)  [unwired: 10 in, 5 out]
        n274 = property on="Total Routine Time" class="Slide (strict)"("Scale.Maximum"=w550) -> ()  [unwired: 2 in, 2 out]
        n275 = Seconds To Date/Time(time stamp (now)=w552) -> (date time rec=w554:T2)  [unwired: 1 in]
        n276 = case shown="False" w549 {
          frame False {
            n277 = flat-sequence {
              frame #0 {
                w555 = FALSE
                w556 = TRUE
                n278 = local write "Output"(w556) -> ()
                n279 = local write "Start Acquisition"(w556) -> ()
                n280 = local write "Play Sound"(w556) -> ()
                n281 = local write "Stop Acquisition"(w555) -> ()
                n282 = local write "BIO Connect"(w555) -> ()
              }
              frame #1 {
                n283 = local write "Buffer"(TRUE) -> ()
              }
            }
          }
          frame True {
            # "Routine done. Save."
            n284 = flat-sequence {
              frame #0 {
                n285 = local write "Buffer"(FALSE) -> ()
              }
              frame #1 {
                w560 = FALSE
                n286 = local write "Stop Acquisition"(TRUE) -> ()
                n287 = local write "Output"(w560) -> ()
                n288 = local write "Start Acquisition"(w560) -> ()
                n289 = local write "Play Sound"(w560) -> ()
              }
              frame #2 {
                n290 = local write "Save"(TRUE) -> ()
              }
              frame #3 {
                n291 = Wait (ms)(milliseconds to wait=500) -> ()  [unwired: 1 out]
              }
              frame #4 {
                n292 = local write "Flush"(TRUE) -> ()
              }
              frame #5 {
                n293 = local write "Flush"(FALSE) -> ()
                n294 = local write "Save"(FALSE) -> ()
              }
              frame #6 {
                n295 = local write "Routine Selection"(enum16{"Default"}."Default") -> ()
              }
            }
          }
        }
      }
      frame "Routine 5b" {
        w575 = 300.0  # Routine Time
        # "Attention"
        n296 = local read "Output"() -> (w570:bool)
        n297 = Not(x=w570) -> (.not. x?=w571:bool)
        n298 = call "Elapsed Time6"("Time Target (s)"=w575, "Reset"=w571) -> ("Get Start Time (s)"=w574:dbl, "Elapsed Time (s)"=w569:dbl, "Time has Elapsed"=w572:bool)  [unwired: 10 in, 5 out]
        n299 = property on="Total Routine Time" class="Slide (strict)"("Scale.Maximum"=w575) -> ()  [unwired: 2 in, 2 out]
        n300 = Seconds To Date/Time(time stamp (now)=w574) -> (date time rec=w573:T2)  [unwired: 1 in]
        n301 = case shown="False" w572 {
          frame False {
            # "Routine Not Done. Continue buffering."
            n302 = flat-sequence {
              tunnel: "OpenHTML" -> [w580]
              frame #0 {
                w579 = FALSE
                w578 = TRUE
                n303 = case shown="True" w580 {
                  frame False {
                  }
                  frame True {
                    n304 = local write "OpenHTML"(FALSE) -> ()
                    n305 = call-poly <vilib>:"Open URL in Default Browser.vi"("URL"="\"C:\\Users\\tbc38\\Documents\\AttentionTest\\mackworth\\vigilanceTest.html\"") -> ()  [unwired: 5 in, 2 out]
                  }
                }
                n306 = local write "Stop Acquisition"(w579) -> ()
                n307 = local write "Play Sound"(w578) -> ()
                n308 = local write "Output"(w578) -> ()
                n309 = local write "Start Acquisition"(w578) -> ()
                n310 = local write "BIO Connect"(w579) -> ()
              }
              frame #1 {
                n311 = local write "Buffer"(TRUE) -> ()
              }
            }
          }
          frame True {
            # "Routine done. Save."
            n312 = flat-sequence {
              frame #0 {
                n313 = local write "Buffer"(FALSE) -> ()
              }
              frame #1 {
                w585 = FALSE
                n314 = local write "Play Sound"(w585) -> ()
                n315 = local write "Output"(w585) -> ()
                n316 = local write "Start Acquisition"(w585) -> ()
                n317 = local write "Stop Acquisition"(TRUE) -> ()
              }
              frame #2 {
                n318 = local write "Save"(TRUE) -> ()
              }
              frame #3 {
                n319 = Wait (ms)(milliseconds to wait=500) -> ()  [unwired: 1 out]
              }
              frame #4 {
                n320 = local write "Flush"(TRUE) -> ()
              }
              frame #5 {
                n321 = local write "Save"(FALSE) -> ()
                n322 = local write "Flush"(FALSE) -> ()
              }
              frame #6 {
                n323 = local write "Routine Selection"(enum16{"Default"}."Default") -> ()
              }
            }
          }
        }
      }
    }
    "Current Routine" <- w368
    "Current Instruction" <- w362
    "Next Instruction" <- w365
    "Total Routine Time" <- w363
    "Elapsed Time" <- w364
    "Start Time" <- w361
  }
  n324 = To Unsigned Long Integer(number=w3) -> (unsigned 32bit integer=w17:u32)
  n325 = Initialize Array(0.0, w4, w17) -> (w19:dbl[][])
  n326 = property class="niUSRP"(reference=w127, error in=w128, "Carrier Frequency"="Ch3&4 carrier frequency [Hz] 2", "Bandwidth"=5000000.0 ("Configuration:Bandwidth")) -> (reference out=w98:refnum<k15>, error out=w97:errorcluster)
  n327 = Obtain Queue(max queue size (-1, unlimited)=-1, name (unnamed)="BIOPAC View", element data type=w19) -> (queue out=w10:refnum<queue>)  [unwired: 2 in, 2 out]
  n328 = property class="niUSRP"(reference=w193, error in=w194, "Carrier Frequency"="Ch1&2 carrier frequency [Hz]", "Bandwidth"=5000000.0 ("Configuration:Bandwidth")) -> (reference out=w164:refnum<k15>, error out=w163:errorcluster)
  n329 = while {
    tunnel: w10 -> [w611]
    shift-right: [w605] -> _
    shift-left: dbl[] [] -> [w606]
    shift-right: [w603] -> _
    shift-left: dbl[] [] -> [w604]
    shift-right: [w602] -> _
    shift-left: dbl[] [] -> [w601]
    shift-right: [w599] -> _
    shift-left: dbl[] [] -> [w600]
    stop <- FALSE stop-if-true
    # "SHOW/VIEWING"
    n330 = local read "ACQ ms"() -> (w594:dbl)
    n331 = local read "Receiving"() -> (w593:bool)
    n332 = Get Queue Status(queue=w611) -> (# elements in queue=w609:i32)  [unwired: 2 in, 7 out]
    "# BIOViewQ2" <- w609
    n333 = Wait (ms)(milliseconds to wait=w594) -> ()  [unwired: 1 out]
    n334 = And(x="Show BIO", y=w593) -> (x .and. y?=w607:bool)
    n335 = case shown="True" w607 {
      tunnel: w611 -> [_ w626]
      tunnel: w609 -> [_ w625]
      tunnel: w606 -> [_ w623]
      tunnel: [w612 w622] -> w605
      tunnel: w604 -> [_ w620]
      tunnel: [w612 w619] -> w603
      tunnel: [w612 w618] -> w602
      tunnel: w601 -> [_ w616]
      tunnel: [w612 w615] -> w599
      tunnel: w600 -> [_ w613]
      frame False {
        w612 = dbl[] []
      }
      frame True {
        n336 = for {
          N: w625 -> [_]
          tunnel: [w635] -> w621 mode=concatenating
          tunnel: [w632] -> w617 mode=concatenating
          tunnel: [w631] -> w614 mode=concatenating
          tunnel: w626 -> [w628]
          tunnel: [w627] -> w624 mode=concatenating
          n337 = Dequeue Element(queue=w628) -> (element=w629:dbl[][])  [unwired: 2 in, 3 out]
          n338 = Index Array(array=w629, index (row)=0) -> (element=w631:dbl[])  [unwired: 1 in]
          n339 = Index Array(array=w629, index (row)=1) -> (element=w632:dbl[])  [unwired: 1 in]
          n340 = Index Array(array=w629, index (row)=2) -> (element=w635:dbl[])  [unwired: 1 in]
          n341 = Index Array(array=w629, index (row)=3) -> (element=w627:dbl[])  [unwired: 1 in]
        }
        n342 = Build Array (concatenate)(w613, w614) -> (w615:dbl[])
        n343 = Build Array (concatenate)(w616, w617) -> (w618:dbl[])
        n344 = Build Array (concatenate)(w620, w621) -> (w619:dbl[])
        n345 = Build Array (concatenate)(w623, w624) -> (w622:dbl[])
      }
    }
    "Array 1 View" <- w599
    "Array 2 View" <- w602
    "Array 3 View" <- w603
    "Array 4 View" <- w605
    n346 = local read "# ACQ cycles"() -> (w595:i32)
    n347 = Array Size(array=w599) -> (size(s)=w598:i32)
    "View Array Size" <- w598
    n348 = Divide(x=w598, y=w594) -> (x/y=w597:dbl)
    "# Elements in Array" <- w597
    n349 = Subtract(x=w595, y=w597) -> (x-y=→"ACQ -# Elements":dbl)
  }
  n350 = property class="niUSRP"(reference=w98, error in=w97, "Active Channel"="0", "Gain"="Rx2 Gain 1", "Active Antenna"=w85) -> (reference out=w102:refnum<k15>, error out=w101:errorcluster)
  n351 = property class="niUSRP" props=["Active Channel", "Gain", "Active Antenna", "Bandwidth"](reference=w164, error in=w163, "Active Channel"="0", "Gain"="Rx1 Gain 1", "Active Antenna"=w86) -> (reference out=w168:refnum<k15>, error out=w167:errorcluster)  [unwired: 1 out]
  n352 = To Unsigned Long Integer(number=w3) -> (unsigned 32bit integer=w6:u32)
  n353 = Initialize Array(0.0, w4, w6) -> (w8:dbl[][])
  n354 = Obtain Queue(max queue size (-1, unlimited)=-1, name (unnamed)="BIOPAC Buffer", element data type=w8) -> (queue out=w2:refnum<queue>)  [unwired: 2 in, 2 out]
  n355 = while {
    tunnel: w10 -> [w637]
    tunnel: w2 -> [w639]
    stop <- FALSE stop-if-true
    # "START ACQUISITION"
    n356 = local read "Connected"() -> (w644:bool)
    n357 = local read "Receiving"() -> (w642:bool)
    n358 = Not(x=w642) -> (.not. x?=w643:bool)
    n359 = And(x=w644, y=w643) -> (x .and. y?=w645:bool)
    n360 = And(x="Start Acquisition", y=w645) -> (x .and. y?=w646:bool)
    n361 = case shown="True" w646 {
      tunnel: w637 -> [_ w651]
      tunnel: w639 -> [_ w650]
      frame False {
      }
      frame True {
        n362 = flat-sequence {
          tunnel: [w656] -> w649
          tunnel: w649 -> [w660]
          tunnel: [w660] -> w648
          tunnel: w648 -> [w662]
          tunnel: [w662] -> w652
          tunnel: w652 -> [w665]
          tunnel: w651 -> [w664]
          tunnel: w650 -> [w663]
          frame #0 {
            n363 = dll-call lib="C:/Program Files (x86)/BIOPAC Systems, Inc/BIOPAC Hardware API 2.2 Education/x64/mpdev.dll" fn="startMPAcqDaemon" label="start Acq Daemon"() -> ()  [unwired: 4 in, 2 out]
            n364 = local write "Start Acquisition"(FALSE) -> ()
            n365 = local write "Stop Acquisition"(FALSE) -> ()
            n366 = local write "Receiving"(TRUE) -> ()
          }
          frame #1 {
            w657 = u32 1  # MPSUCCESS
            n367 = dll-call lib="C:/Program Files (x86)/BIOPAC Systems, Inc/BIOPAC Hardware API 2.2 Education/x64/mpdev.dll" fn="startAcquisition" label="start Acquisition"() -> ("return type"=w658:u32)  [unwired: 3 in, 2 out]
            n368 = Equal?(x=w658, y=w657) -> (x = y?=w656:bool)
          }
          frame #2 {
            n369 = local write "Acq Started"(TRUE) -> ()
          }
          frame #3 {
            n370 = local read "ACQ ms"() -> (w661:dbl)
            n371 = Wait (ms)(milliseconds to wait=w661) -> ()  [unwired: 1 out]
          }
          frame #4 {
            n372 = local read "Sample Rate"() -> (w670:dbl)
            n373 = local read "# Channels"() -> (w668:dbl)
            n374 = local read "ACQ ms"() -> (w669:dbl)
            n375 = Reciprocal(x=w670) -> (1/x=w673:dbl)
            n376 = Multiply(x=w673, y=w669) -> (x*y=w671:dbl)
            n377 = Multiply(x=w671, y=w668) -> (x*y=w666:dbl)
            "Receive Total Size" <- w666
            n378 = Initialize Array(0.0, w666) -> (w667:dbl[])
            n379 = case shown="True" w665 {
              tunnel: w667 -> [_ w678]
              tunnel: w666 -> [_ w677]
              tunnel: w664 -> [_ w676]
              tunnel: w663 -> [_ w674]
              frame False {
              }
              frame True {
                n380 = while {
                  tunnel: w678 -> [w704]
                  tunnel: w677 -> [w703]
                  tunnel: w676 -> [w679]
                  shift-right: [w690] -> _
                  shift-left: 0 -> [w691]
                  tunnel: w674 -> [w683]
                  stop <- w686 stop-if-true
                  w701 = u32 1  # MPSUCCESS
                  n381 = Add(x=w691, y=1) -> (x+y=w690:i32)
                  "# ACQ cycles" <- w690
                  n382 = dll-call lib="C:/Program Files (x86)/BIOPAC Systems, Inc/BIOPAC Hardware API 2.2 Education/x64/mpdev.dll" fn="receiveMPData"("value"=w704, "bytetoread"=w703, "bytesread"=0) -> ("return type"=w702:i32, "value"=w696:dbl[], "bytetoread"=→"Bytes To Read":u32, "bytesread"=→"Bytes Read":i32)  [unwired: 3 in, 2 out]
                  n383 = Decimate 1D Array(w696) -> (w697:dbl[], w698:dbl[], w699:dbl[], w695:dbl[])
                  n384 = Equal?(x=w702, y=w701) -> (x = y?=w685:bool)
                  n385 = Build Array(w697, w698, w699, w695) -> (w680:dbl[][])
                  n386 = local read "Show BIO"() -> (w681:bool)
                  n387 = local write "Receive Success"(w685) -> ()
                  n388 = case shown="True" w681 {
                    tunnel: w680 -> [_ w706]
                    tunnel: w679 -> [_ w705]
                    frame False {
                    }
                    frame True {
                      n389 = Enqueue Element(queue=w705, element=w706) -> ()  [unwired: 2 in, 3 out]
                    }
                  }
                  n390 = local read "Buffer"() -> (w684:bool)
                  n391 = case shown="True" w684 {
                    tunnel: w680 -> [_ w708]
                    tunnel: w683 -> [_ w707]
                    frame False {
                    }
                    frame True {
                      n392 = Enqueue Element(queue=w707, element=w708) -> ()  [unwired: 2 in, 3 out]
                    }
                  }
                  n393 = Get Queue Status(queue=w683) -> (# elements in queue=w682:i32)  [unwired: 2 in, 7 out]
                  n394 = local write "# BIO Buffer"(w682) -> ()
                  n395 = local read "Stop Acquisition"() -> (w686:bool)
                  n396 = local read "ACQ ms"() -> (w687:dbl)
                  n397 = Subtract(x=w687, y=0.0) -> (x-y=w694:dbl)
                  n398 = Wait (ms)(milliseconds to wait=w694) -> ()  [unwired: 1 out]
                }
              }
            }
          }
          frame #5 {
            n399 = local write "Receiving"(FALSE) -> ()
            n400 = local write "Acq Started"(FALSE) -> ()
          }
        }
      }
    }
    n401 = Get Queue Status(queue=w637) -> (# elements in queue=→"# BIO View Q":i32)  [unwired: 2 in, 7 out]
    n402 = Get Queue Status(queue=w639) -> (# elements in queue=→"# BIO Buffer":i32)  [unwired: 2 in, 7 out]
  }
  n403 = property class="niUSRP"(reference=w102, error in=w101, "Active Channel"="1", "Gain"="Rx2 Gain 2", "Active Antenna"=w85) -> (reference out=w130:refnum<k15>, error out=w129:errorcluster)
  n404 = call <instrlib>:"niUSRP Open Tx Session.vi"("device names"=w150, "error in (no error)"=w129) -> ("session handle out"=w137:refnum<k15>, "error out"=w136:errorcluster)  [unwired: 12 in]
  n405 = property class="niUSRP"(reference=w137, error in=w136, "Enabled Channels"="0,1" ("Configuration:Enabled Channels")) -> (reference out=w125:refnum<k15>, error out=w124:errorcluster)
  n406 = property class="niUSRP"(reference=w125, error in=w124, "IQ Rate"="Tx IQ Rate 2") -> (reference out=w119:refnum<k15>, error out=w120:errorcluster, "IQ Rate"=w118:dbl)
  n407 = property class="niUSRP" props=["Model", "Reference Frequency Source", "Timebase Clock Source"](reference=w119, error in=w120, "Reference Frequency Source"="RefIn" ("Clocking and Synchronization:Reference Frequency Source"), "Timebase Clock Source"="PpsIn" ("Clocking and Synchronization:Timebase Clock Source")) -> (reference out=w121:refnum<k15>, error out=w122:errorcluster)  [unwired: 1 out]
  n408 = property class="niUSRP"(reference=w121, error in=w122, "Carrier Frequency"="Ch3&4 carrier frequency [Hz] 2") -> (reference out=w92:refnum<k15>, error out=w91:errorcluster)
  n409 = property class="niUSRP"(reference=w92, error in=w91, "Active Channel"="0", "Gain"="Tx2 Gain 1", "Active Antenna"=w114) -> (reference out=w96:refnum<k15>, error out=w95:errorcluster)
  n410 = property class="niUSRP"(reference=w96, error in=w95, "Active Channel"="1", "Gain"="Tx2 Gain 2", "Active Antenna"=w114) -> (reference out=w116:refnum<k15>, error out=w117:errorcluster)
  n411 = property class="niUSRP"(reference=w168, error in=w167, "Active Channel"="1", "Gain"="Rx1 Gain 2", "Active Antenna"=w86) -> (reference out=w196:refnum<k15>, error out=w195:errorcluster)
  n412 = call <instrlib>:"niUSRP Open Tx Session.vi"("device names"=w216, "error in (no error)"=w195) -> ("session handle out"=w203:refnum<k15>, "error out"=w202:errorcluster)  [unwired: 12 in]
  n413 = property class="niUSRP"(reference=w203, error in=w202, "Enabled Channels"="0,1" ("Configuration:Enabled Channels")) -> (reference out=w191:refnum<k15>, error out=w190:errorcluster)
  n414 = property class="niUSRP"(reference=w191, error in=w190, "IQ Rate"="Tx IQ Rate 1") -> (reference out=w185:refnum<k15>, error out=w186:errorcluster, "IQ Rate"=w184:dbl)
  n415 = property class="niUSRP" props=["Model", "Reference Frequency Source", "Timebase Clock Source"](reference=w185, error in=w186, "Reference Frequency Source"="RefIn" ("Clocking and Synchronization:Reference Frequency Source"), "Timebase Clock Source"="PpsIn" ("Clocking and Synchronization:Timebase Clock Source")) -> (reference out=w187:refnum<k15>, error out=w188:errorcluster)  [unwired: 1 out]
  n416 = property class="niUSRP"(reference=w187, error in=w188, "Carrier Frequency"="Ch1&2 carrier frequency [Hz]") -> (reference out=w158:refnum<k15>, error out=w157:errorcluster)
  n417 = property class="niUSRP"(reference=w158, error in=w157, "Active Channel"="0", "Gain"="Tx1 Gain 1", "Active Antenna"=w180) -> (reference out=w162:refnum<k15>, error out=w161:errorcluster)
  n418 = property class="niUSRP"(reference=w162, error in=w161, "Active Channel"="1", "Gain"="Tx1 Gain 2", "Active Antenna"=w180) -> (reference out=w182:refnum<k15>, error out=w183:errorcluster)
  n419 = while {
    stop <- FALSE stop-if-true
    # "DISCONNECT"
    n420 = Wait (ms)(milliseconds to wait=500) -> ()  [unwired: 1 out]
    n421 = case shown="True" "Disconnect" {
      frame False {
      }
      frame True {
        w714 = FALSE
        n422 = dll-call lib="C:/Program Files (x86)/BIOPAC Systems, Inc/BIOPAC Hardware API 2.2 Education/x64/mpdev.dll" fn="disconnectMPDev" label="disconnect"() -> ()  [unwired: 4 in, 2 out]
        n423 = local write "Disconnect"(w714) -> ()
        n424 = local write "Disconnected"(TRUE) -> ()
        n425 = local write "Connected"(w714) -> ()
      }
    }
  }
  n426 = while {
    stop <- FALSE stop-if-true
    n427 = local read "Output"() -> (w717:bool)
    n428 = Wait (ms)(milliseconds to wait=10.0) -> ()  [unwired: 1 out]
    n429 = case shown="True" w717 {
      tunnel: [w723 "Channel 1 Tone Amplitude"] -> w721
      tunnel: [w723 "Channel 2 Tone Amplitude"] -> w720
      tunnel: [w723 "Channel 3 Tone Amplitude"] -> w719
      tunnel: [w723 "Channel 4 Tone Amplitude"] -> w718
      frame False {
        w723 = 0.0 ("Channel 1\nTone Amplitude")
      }
      frame True {
      }
    }
    "Ch1 Amplitude" <- w721
    "Ch2 Amplitude" <- w720
    "Ch3 Amplitude" <- w719
    "Ch4 Amplitude" <- w718
  }
  n430 = call <instrlib>:"niUSRP Commit.vi"("session handle"=w116, "error in (no error)"=w117) -> ("session handle out"=w152:refnum<k15>, "error out"=w153:errorcluster)  [unwired: 12 in]
  n431 = call <instrlib>:"niUSRP Commit.vi"("session handle"=w182, "error in (no error)"=w183) -> ("session handle out"=w218:refnum<k15>, "error out"=w219:errorcluster)  [unwired: 12 in]
  n432 = Merge Errors(w129, w153) -> (w144:errorcluster)
  n433 = Merge Errors(w195, w219) -> (w210:errorcluster)
  n434 = call <instrlib>:"niUSRP Set Time.vi"("session handle"=w130, "apply timestamp"=w142, "timestamp"=T4 {"whole seconds"=0, "fractional seconds"=0.0}, "error in (no error)"=w144) -> ("session handle out"=w146:refnum<k15>, "error out"=w145:errorcluster)  [unwired: 10 in]
  n435 = call <instrlib>:"niUSRP Initiate.vi"("session handle"=w146, "error in (no error)"=w145) -> ("session handle out"=w156:refnum<k15>, "error out"=w84:errorcluster)  [unwired: 12 in]
  n436 = while {
    tunnel: w118 -> [w746]
    tunnel: w84 -> [w741]
    stop <- FALSE stop-if-true
    # "Generate I and Q waveforms."
    n437 = Bundle By Name(cluster=cluster{"Fs":dbl, "#s":dbl} {"Fs"=1000.0, "#s"=1000.0} ("sampling info"), "Fs"=w746, "#s"="Waveform Size 2") -> (w747:cluster{"Fs":dbl, "#s":dbl})
    n438 = Wait (ms)(milliseconds to wait=u32 500) -> ()  [unwired: 1 out]
    n439 = local read "Ch3 Amplitude"() -> (w737:dbl)
    n440 = local read "Ch4 Amplitude"() -> (w736:dbl)
    n441 = call <vilib>:"Sine Waveform.vi"("sampling info"=w747, "error in (no error)"=w741, "phase"=90.0, "amplitude"=w737, "frequency"="Channel 3 Tone Frequency") -> ("error out"=w742:errorcluster, "signal out"=w760:waveform(dbl))  [unwired: 5 in]
    n442 = call <vilib>:"Sine Waveform.vi"("sampling info"=w747, "error in (no error)"=w741, "amplitude"=w737, "frequency"="Channel 3 Tone Frequency") -> ("error out"=w743:errorcluster, "signal out"=w761:waveform(dbl))  [unwired: 6 in]
    n443 = call <vilib>:"Sine Waveform.vi"("sampling info"=w747, "error in (no error)"=w741, "phase"=90.0, "amplitude"=w736, "frequency"="Channel 4 Tone Frequency") -> ("error out"=w744:errorcluster, "signal out"=w751:waveform(dbl))  [unwired: 5 in]
    n444 = call <vilib>:"Sine Waveform.vi"("sampling info"=w747, "error in (no error)"=w741, "amplitude"=w736, "frequency"="Channel 4 Tone Frequency") -> ("error out"=w745:errorcluster, "signal out"=w750:waveform(dbl))  [unwired: 6 in]
    n445 = Merge Errors(w742, w743, w744, w745) -> ()  [unwired: 1 out]
    n446 = Build Array(w760, w761, w751, w750) -> (→"Tx2 Waveform Graph":waveform(dbl)[])
    n447 = Unbundle By Name(w760) -> ("Y"=w759:dbl[])
    n448 = Unbundle By Name(w761) -> ("Y"=w758:dbl[])
    n449 = Unbundle By Name(w751) -> ("Y"=w754:dbl[])
    n450 = Unbundle By Name(w750) -> ("Y"=w753:dbl[])
    n451 = Re/Im To Complex(1:w758, 2:w759) -> (0:w749:cdb[])
    n452 = Re/Im To Complex(1:w753, 2:w754) -> (0:w748:cdb[])
    n453 = Build Array(w749, w748) -> (→"Tx2 Waveform":cdb[][])
    n454 = local read "Tx2 Waveform"() -> (w734:cdb[][])
    n455 = local read "Tx2 Waveform"() -> (w730:cdb[][])
    n456 = Index Array(array=w734, index (row)=0) -> (element=w733:cdb[])  [unwired: 1 in]
    n457 = Index Array(array=w730, index (row)=1) -> (element=w729:cdb[])  [unwired: 1 in]
    n458 = Complex To Polar(r * e^(i*theta)=w733) -> (theta=→"Tx ch3  ph":dbl[])  [unwired: 1 out]
    n459 = Complex To Polar(r * e^(i*theta)=w729) -> (theta=→"Tx ch4 ph":dbl[])  [unwired: 1 out]
  }
  n460 = call <instrlib>:"niUSRP Set Time.vi"("session handle"=w196, "apply timestamp"=w208, "timestamp"=T4 {"whole seconds"=0, "fractional seconds"=0.0}, "error in (no error)"=w210) -> ("session handle out"=w212:refnum<k15>, "error out"=w211:errorcluster)  [unwired: 10 in]
  n461 = call <instrlib>:"niUSRP Initiate.vi"("session handle"=w212, "error in (no error)"=w211) -> ("session handle out"=w222:refnum<k15>, "error out"=w83:errorcluster)  [unwired: 12 in]
  n462 = while {
    tunnel: w184 -> [w783]
    tunnel: w83 -> [w775]
    stop <- FALSE stop-if-true
    # "Generate I and Q waveforms."
    n463 = Wait (ms)(milliseconds to wait=u32 500) -> ()  [unwired: 1 out]
    n464 = Bundle By Name(cluster=cluster{"Fs":dbl, "#s":dbl} {"Fs"=1000.0, "#s"=1000.0} ("sampling info"), "Fs"=w783, "#s"="Waveform Size 1") -> (w784:cluster{"Fs":dbl, "#s":dbl})
    n465 = local read "Ch1 Amplitude"() -> (w774:dbl)
    n466 = local read "Ch2 Amplitude"() -> (w773:dbl)
    n467 = call <vilib>:"Sine Waveform.vi"("sampling info"=w784, "error in (no error)"=w775, "phase"=90.0, "amplitude"=w774, "frequency"="Channel 1 Tone Frequency") -> ("error out"=w779:errorcluster, "signal out"=w797:waveform(dbl))  [unwired: 5 in]
    n468 = call <vilib>:"Sine Waveform.vi"("sampling info"=w784, "error in (no error)"=w775, "amplitude"=w774, "frequency"="Channel 1 Tone Frequency") -> ("error out"=w780:errorcluster, "signal out"=w798:waveform(dbl))  [unwired: 6 in]
    n469 = call <vilib>:"Sine Waveform.vi"("sampling info"=w784, "error in (no error)"=w775, "phase"=90.0, "amplitude"=w773, "frequency"="Channel 2 Tone Frequency") -> ("error out"=w781:errorcluster, "signal out"=w788:waveform(dbl))  [unwired: 5 in]
    n470 = call <vilib>:"Sine Waveform.vi"("sampling info"=w784, "error in (no error)"=w775, "amplitude"=w773, "frequency"="Channel 2 Tone Frequency") -> ("error out"=w782:errorcluster, "signal out"=w787:waveform(dbl))  [unwired: 6 in]
    n471 = Merge Errors(w779, w780, w781, w782) -> ()  [unwired: 1 out]
    n472 = Build Array(w797, w798, w788, w787) -> (→"Tx1 Waveform Graph":waveform(dbl)[])
    n473 = local read "Tx1 Waveform"() -> (w771:cdb[][])
    n474 = local read "Tx1 Waveform"() -> (w766:cdb[][])
    n475 = Unbundle By Name(w797) -> ("Y"=w796:dbl[])
    n476 = Unbundle By Name(w798) -> ("Y"=w795:dbl[])
    n477 = Unbundle By Name(w788) -> ("Y"=w791:dbl[])
    n478 = Unbundle By Name(w787) -> ("Y"=w790:dbl[])
    n479 = Re/Im To Complex(1:w795, 2:w796) -> (0:w786:cdb[])
    n480 = Re/Im To Complex(1:w790, 2:w791) -> (0:w785:cdb[])
    n481 = Build Array(w786, w785) -> (→"Tx1 Waveform":cdb[][])
    n482 = Index Array(array=w766, index (row)=0) -> (element=w767:cdb[])  [unwired: 1 in]
    n483 = Index Array(array=w771, index (row)=1) -> (element=w770:cdb[])  [unwired: 1 in]
    n484 = Complex To Polar(r * e^(i*theta)=w770) -> (theta=→"Tx ch2  ph":dbl[])  [unwired: 1 out]
    n485 = Complex To Polar(r * e^(i*theta)=w767) -> (theta=→"Tx ch1  ph":dbl[])  [unwired: 1 out]
  }
  n486 = local read "Waveform Size 2"() -> (w63:dbl)
  n487 = local read "Waveform Size 1"() -> (w73:dbl)
  n488 = Initialize Array(cdb 0.0+0.0i ("element"), 2 ("dimension size"), w63) -> (w65:cdb[][])
  n489 = Obtain Queue(max queue size (-1, unlimited)=-1, name (unnamed)="Rx2Queue", element data type=w65) -> (queue out=w61:refnum<queue>)  [unwired: 2 in, 2 out]
  n490 = Initialize Array(cdb 0.0+0.0i ("element"), 2 ("dimension size"), w73) -> (w70:cdb[][])
  n491 = Obtain Queue(max queue size (-1, unlimited)=-1, name (unnamed)="Rx1Queue", element data type=w70) -> (queue out=w62:refnum<queue>)  [unwired: 2 in, 2 out]
  n492 = while {
    tunnel: w61 -> [w802]
    stop <- FALSE stop-if-true
    n493 = Wait (ms)(milliseconds to wait=u32 200) -> ()  [unwired: 1 out]
    n494 = case shown="True" "Dis2" {
      tunnel: w802 -> [_ w808]
      frame False {
        n495 = Wait (ms)(milliseconds to wait=u32 500) -> ()  [unwired: 1 out]
      }
      frame True {
        n496 = Preview Queue Element(queue=w808) -> (element=w809:cdb[][])  [unwired: 2 in, 3 out]
        n497 = for {
          tunnel: w809 -> [w815] mode=indexing
          shift-right: [w812] -> w807
          shift-left: dbl[][] [] -> [w811]
          n498 = Complex To Re/Im(x + iy=w815) -> (x=w814:dbl[], y=w813:dbl[])
          n499 = Build Array (concatenate)(w811, w814, w813) -> (w812:dbl[][])
        }
        "IQ Graph 2" <- w807
      }
    }
  }
  n500 = while {
    tunnel: w156 -> [w826]
    tunnel: w84 -> [w825]
    tunnel: [w821] -> w111
    tunnel: [w824] -> w108
    shift-right: [w816] -> _
    shift-left: w61 -> [w817]
    stop <- w820 stop-if-true
    # "Rx on both channels"
    n501 = local read "Waveform Size 2"() -> (w819:dbl)
    n502 = call-poly <instrlib>:"niUSRP Fetch Rx Data (poly).vi"("session handle"=w826, "number of samples"=w819, "error in (no error)"=w825) -> ("session handle out"=w824:refnum<k15>, "data"=w818:cdb[][], "error out"=w821:errorcluster)  [unwired: 9 in, 1 out]
    n503 = Enqueue Element(queue=w817, element=w818) -> (queue out=w816:refnum<queue>)  [unwired: 2 in, 2 out]
    n504 = Unbundle By Name(w821) -> ("status"=w823:bool)
    n505 = Or(x=w823, y="Stop 2") -> (x .or. y?=w820:bool)
  }
  n506 = while {
    tunnel: w152 -> [w834]
    tunnel: w84 -> [w833]
    tunnel: [w831] -> w113
    tunnel: [w829] -> w106
    stop <- w830 stop-if-true
    # "Tx on both channels"
    n507 = local read "Tx2 Waveform"() -> (w827:cdb[][])
    n508 = local read "Stop 2"() -> (w828:bool)
    n509 = call-poly <instrlib>:"niUSRP Write Tx Data (poly).vi"("session handle"=w834, "data"=w827, "end of data?"=w828, "error in (no error)"=w833) -> ("session handle out"=w829:refnum<k15>, "error out"=w831:errorcluster)  [unwired: 10 in]
    n510 = Unbundle By Name(w831) -> ("status"=w832:bool)
    n511 = Compound Arithmetic op=OR(w832, w828) -> (w830:bool)
  }
  n512 = while {
    tunnel: w62 -> [w836]
    stop <- FALSE stop-if-true
    n513 = Wait (ms)(milliseconds to wait=u32 200) -> ()  [unwired: 1 out]
    n514 = case shown="True" "Dis1" {
      tunnel: w836 -> [_ w840]
      frame False {
        n515 = Wait (ms)(milliseconds to wait=u32 500) -> ()  [unwired: 1 out]
      }
      frame True {
        n516 = Preview Queue Element(queue=w840) -> (element=w842:cdb[][])  [unwired: 2 in, 3 out]
        n517 = for {
          tunnel: w842 -> [w848] mode=indexing
          shift-right: [w845] -> w841
          shift-left: dbl[][] [] -> [w844]
          n518 = Complex To Re/Im(x + iy=w848) -> (x=w847:dbl[], y=w846:dbl[])
          n519 = Build Array (concatenate)(w844, w847, w846) -> (w845:dbl[][])
        }
        "IQ Graph" <- w841
      }
    }
  }
  n520 = while {
    tunnel: w222 -> [w859]
    tunnel: w83 -> [w858]
    tunnel: [w854] -> w177
    tunnel: [w857] -> w174
    shift-right: [w849] -> _
    shift-left: w62 -> [w851]
    stop <- w853 stop-if-true
    # "Rx on both channels"
    n521 = local read "Waveform Size 1"() -> (w852:dbl)
    n522 = call-poly <instrlib>:"niUSRP Fetch Rx Data (poly).vi"("session handle"=w859, "number of samples"=w852, "error in (no error)"=w858) -> ("session handle out"=w857:refnum<k15>, "data"=w850:cdb[][], "error out"=w854:errorcluster)  [unwired: 9 in, 1 out]
    n523 = Enqueue Element(queue=w851, element=w850) -> (queue out=w849:refnum<queue>)  [unwired: 2 in, 2 out]
    n524 = Unbundle By Name(w854) -> ("status"=w856:bool)
    n525 = Or(x=w856, y="Stop") -> (x .or. y?=w853:bool)
  }
  n526 = while {
    tunnel: w218 -> [w867]
    tunnel: w83 -> [w866]
    tunnel: [w864] -> w179
    tunnel: [w862] -> w172
    stop <- w863 stop-if-true
    # "Tx on both channels"
    n527 = local read "Tx1 Waveform"() -> (w860:cdb[][])
    n528 = local read "Stop"() -> (w861:bool)
    n529 = call-poly <instrlib>:"niUSRP Write Tx Data (poly).vi"("session handle"=w867, "data"=w860, "end of data?"=w861, "error in (no error)"=w866) -> ("session handle out"=w862:refnum<k15>, "error out"=w864:errorcluster)  [unwired: 10 in]
    n530 = Unbundle By Name(w864) -> ("status"=w865:bool)
    n531 = Compound Arithmetic op=OR(w865, w861) -> (w863:bool)
  }
  n532 = flat-sequence {
    tunnel: [w869] -> w112
    tunnel: w113 -> [w869]
    tunnel: [w868] -> w107
    tunnel: w106 -> [w868]
    frame #0 {
      n533 = local write "Stop 2"(TRUE ("STOP")) -> ()
    }
  }
  n534 = flat-sequence {
    tunnel: [w872] -> w178
    tunnel: w179 -> [w872]
    tunnel: [w871] -> w173
    tunnel: w172 -> [w871]
    frame #0 {
      n535 = local write "Stop"(TRUE ("STOP")) -> ()
    }
  }
  n536 = flat-sequence {
    tunnel: [w875] -> w110
    tunnel: w111 -> [w875]
    tunnel: [w874] -> w109
    tunnel: w108 -> [w874]
    frame #0 {
      n537 = local write "Stop 2"(TRUE ("STOP")) -> ()
    }
  }
  n538 = flat-sequence {
    tunnel: [w878] -> w176
    tunnel: w177 -> [w878]
    tunnel: [w877] -> w175
    tunnel: w174 -> [w877]
    frame #0 {
      n539 = local write "Stop"(TRUE ("STOP")) -> ()
    }
  }
  n540 = local read "Rx IQ Rate 1"() -> (w40:dbl)
  n541 = call <instrlib>:"niUSRP Abort.vi"("session handle"=w109, "error in (no error)"=w110) -> ("session handle out"=w149:refnum<k15>, "error out"=w148:errorcluster)  [unwired: 12 in]
  n542 = local read "Waveform Size 1"() -> (w54:dbl)
  n543 = local read "DownSamplingRatio"() -> (w53:i32)
  n544 = call <instrlib>:"niUSRP Close Session.vi"("session handle"=w149, "error in (no error)"=w148) -> ("error out"=w105:errorcluster)  [unwired: 13 in]
  n545 = call <instrlib>:"niUSRP Close Session.vi"("session handle"=w107, "error in (no error)"=w112) -> ("error out"=w104:errorcluster)  [unwired: 13 in]
  n546 = Divide(x=w40, y="DownSamplingRatio1") -> (x/y=→"Sampling Rate":dbl)
  n547 = Divide(x=2000.0, y=2.0) -> (x/y=→"BW/2":dbl)
  n548 = call <instrlib>:"niUSRP Abort.vi"("session handle"=w175, "error in (no error)"=w176) -> ("session handle out"=w215:refnum<k15>, "error out"=w214:errorcluster)  [unwired: 12 in]
  n549 = flat-sequence {
    tunnel: w105 -> [w882]
    tunnel: w104 -> [w881]
    tunnel: [w880] -> w103
    frame #0 {
      n550 = Merge Errors(w882, w881) -> (w880:errorcluster)
      n551 = local write "Stop 2"(FALSE ("STOP")) -> ()
    }
  }
  n552 = Divide(x=w54, y=w53) -> (x/y=w32:dbl)
  n553 = call <instrlib>:"niUSRP Close Session.vi"("session handle"=w215, "error in (no error)"=w214) -> ("error out"=w171:errorcluster)  [unwired: 13 in]
  n554 = call <instrlib>:"niUSRP Close Session.vi"("session handle"=w173, "error in (no error)"=w178) -> ("error out"=w170:errorcluster)  [unwired: 13 in]
  n555 = flat-sequence {
    tunnel: w171 -> [w886]
    tunnel: w170 -> [w885]
    tunnel: [w884] -> w169
    frame #0 {
      n556 = Merge Errors(w886, w885) -> (w884:errorcluster)
      n557 = local write "Stop"(FALSE ("STOP")) -> ()
    }
  }
  n558 = Initialize Array(0.0 ("element"), w33, w32) -> (w55:dbl[][])
  n559 = Initialize Array(0.0 ("element"), w33, w32) -> (w42:dbl[][])
  n560 = Obtain Queue(name (unnamed)="Buffer", element data type=w42) -> (queue out=w41:refnum<queue>)  [unwired: 3 in, 2 out]
  n561 = Obtain Queue(name (unnamed)="ChsQueue", element data type=w55) -> (queue out=w52:refnum<queue>)  [unwired: 3 in, 2 out]
  n562 = while {
    tunnel: w62 -> [w1208]
    tunnel: w61 -> [w1205]
    tunnel: w52 -> [w1165]
    tunnel: w41 -> [w1163]
    tunnel: w2 -> [w1019]
    stop <- FALSE stop-if-true
    w899 = 1 items=["radian in, radian out", "radian in, degree out", "degree in, degree out", "degree in, radian out"] ("phase unit")
    w960 = 1 items=["radian in, radian out", "radian in, degree out", "degree in, degree out", "degree in, radian out"] ("phase unit")
    w1013 = 2 ("order")
    w1042 = Filter_Passband_Type."Bandpass" ("filter type")
    w1071 = Filter_Passband_Type."Bandpass" ("filter type")
    w1012 = Filter_Passband_Type."Bandpass" ("filter type")
    w1108 = Filter_Passband_Type."Bandpass" ("filter type")
    w1014 = 2 ("order")
    # "Tx4 to Rx4 phase"
    # "Tx3 to 4 phase"
    # "Tx2 to Rx4 phase"
    # "Tx1 to Rx4 phase"
    # "Tx4 to Rx3 phase"
    # "Tx3 to 3 phase"
    # "Tx2 to Rx3 phase"
    # "Tx1 to Rx3 phase"
    # "Tx4to Rx2 phase"
    # "Tx3 to Rx2 phase"
    # "Tx2 to Rx2 phase"
    # "Tx1 to Rx2 phase"
    # "Tx4 to Rx1 phase"
    # "Tx3 to Rx1 phase"
    # "Tx2 to Rx1 phase"
    # "Tx1 to Rx1 phase"
    # "Tx4 to Rx4 QueInd_15"
    # "Tx3 to Rx4 QueInd_14"
    # "Tx2 to Rx4 QueInd_13"
    # "Tx1 to Rx4 QueInd_12"
    # "Tx4 to Rx3 QueInd_11"
    # "Tx3 to Rx3 QueInd_10"
    # "Tx2 to Rx3 QueInd_9"
    # "Tx1 to Rx3 QueInd_8"
    # "Tx1 to Rx4 QueInd_12"
    # "Tx2 to Rx4 QueInd_13"
    # "Tx2 to Rx3 QueInd_9"
    # "Tx1 to Rx3 QueInd_8"
    # "Tx4 to Rx2 QueInd_7"
    # "Tx3 to Rx2 QueInd_6"
    # "Tx4 to Rx1 QueInd_3"
    # "Tx3 to Rx1 QueInd_2"
    # "Tx4 to Rx2 QueInd_7"
    # "Tx4 to Rx4 QueInd_15"
    # "Tx3 to Rx2 QueInd_6"
    # "Tx4 to Rx3 QueInd_11"
    # "Tx2 to Rx2 QueInd_5"
    # "Tx2 to Rx2 QueInd_5"
    # "Tx1 to Rx2 QueInd_4"
    # "Tx4 to Rx1 QueInd_3"
    # "Tx3 to Rx1 QueInd_2"
    # "Tx2 to Rx1 QueInd_1"
    # "Tx1 to Rx1 QueInd_0"
    # "Tx2 to Rx1 QueInd_1"
    # "Tx3 to Rx4 QueInd_14"
    # "Tx3 to Rx3 QueInd_10"
    # "Tx1 to Rx2 QueInd_4"
    # "Tx1 to Rx1 QueInd_0"
    # "100 times"
    n563 = Dequeue Element(queue=w1208) -> (element=w1210:cdb[][])  [unwired: 2 in, 3 out]
    n564 = Get Queue Status(queue=w1208) -> (# elements in queue=→"# IQ queue Ch 1":i32)  [unwired: 2 in, 7 out]
    n565 = Get Queue Status(queue=w1205) -> (# elements in queue=→"# IQ queue Ch 2":i32)  [unwired: 2 in, 7 out]
    n566 = Dequeue Element(queue=w1205) -> (element=w1202:cdb[][])  [unwired: 2 in, 3 out]
    n567 = Index Array(array=w1210, index (row)=1) -> (element=w1093:cdb[])  [unwired: 1 in]
    n568 = Index Array(array=w1210, index (row)=0) -> (element=w1111:cdb[])  [unwired: 1 in]
    n569 = Index Array(array=w1202, index (row)=1) -> (element=w1048:cdb[])  [unwired: 1 in]
    n570 = Index Array(array=w1202, index (row)=0) -> (element=w1015:cdb[])  [unwired: 1 in]
    n571 = local read "Channel 2 Tone Frequency"() -> (w1150:dbl)
    n572 = local read "Channel 1 Tone Frequency"() -> (w1162:dbl)
    n573 = local read "Channel 3 Tone Frequency"() -> (w1094:dbl)
    n574 = local read "Channel 4 Tone Frequency"() -> (w1082:dbl)
    n575 = local read "Channel 4 Tone Frequency"() -> (w1110:dbl)
    n576 = local read "Channel 3 Tone Frequency"() -> (w1183:dbl)
    n577 = local read "Channel 3 Tone Frequency"() -> (w1121:dbl)
    n578 = local read "Channel 4 Tone Frequency"() -> (w1130:dbl)
    n579 = local read "Channel 2 Tone Frequency"() -> (w1157:dbl)
    n580 = local read "Channel 2 Tone Frequency"() -> (w1041:dbl)
    n581 = local read "Channel 1 Tone Frequency"() -> (w1199:dbl)
    n582 = local read "Channel 1 Tone Frequency"() -> (w1054:dbl)
    n583 = local read "Rx IQ Rate 1"() -> (w1112:dbl)
    n584 = local read "Channel 1 Tone Frequency"() -> (w1078:dbl)
    n585 = local read "Channel 2 Tone Frequency"() -> (w1059:dbl)
    n586 = local read "Channel 3 Tone Frequency"() -> (w1188:dbl)
    n587 = local read "Channel 4 Tone Frequency"() -> (w1141:dbl)
    n588 = local read "Rx IQ Rate 2"() -> (w1047:dbl)
    n589 = local read "BW/2"() -> (w1109:dbl)
    n590 = local read "BW/2"() -> (w1085:dbl)
    n591 = local read "Rx IQ Rate 1"() -> (w1092:dbl)
    n592 = local read "Rx IQ Rate 2"() -> (w1062:dbl)
    n593 = local read "BW/2"() -> (w1049:dbl)
    n594 = local read "BW/2"() -> (w1060:dbl)
    n595 = Subtract(x=w1094, y=w1085) -> (x-y=w1098:dbl)
    n596 = Subtract(x=w1110, y=w1109) -> (x-y=w1114:dbl)
    n597 = Subtract(x=w1150, y=w1085) -> (x-y=w1148:dbl)
    n598 = Add(x=w1094, y=w1085) -> (x+y=w1099:dbl)
    n599 = Add(x=w1082, y=w1085) -> (x+y=w1083:dbl)
    n600 = Subtract(x=w1082, y=w1085) -> (x-y=w1084:dbl)
    n601 = Subtract(x=w1041, y=w1049) -> (x-y=w1046:dbl)
    n602 = Subtract(x=w1199, y=w1109) -> (x-y=w1200:dbl)
    n603 = Add(x=w1110, y=w1109) -> (x+y=w1115:dbl)
    n604 = Add(x=w1150, y=w1085) -> (x+y=w1149:dbl)
    n605 = Subtract(x=w1157, y=w1109) -> (x-y=w1158:dbl)
    n606 = Subtract(x=w1121, y=w1109) -> (x-y=w1122:dbl)
    n607 = Subtract(x=w1054, y=w1049) -> (x-y=w1055:dbl)
    n608 = Add(x=w1041, y=w1049) -> (x+y=w1045:dbl)
    n609 = Add(x=w1199, y=w1109) -> (x+y=w1201:dbl)
    n610 = Add(x=w1157, y=w1109) -> (x+y=w1159:dbl)
    n611 = Add(x=w1121, y=w1109) -> (x+y=w1123:dbl)
    n612 = Add(x=w1054, y=w1049) -> (x+y=w1056:dbl)
    n613 = Subtract(x=w1162, y=w1085) -> (x-y=w1195:dbl)
    n614 = Add(x=w1162, y=w1085) -> (x+y=w1196:dbl)
    n615 = Subtract(x=w1130, y=w1049) -> (x-y=w1131:dbl)
    n616 = Add(x=w1130, y=w1049) -> (x+y=w1132:dbl)
    n617 = Subtract(x=w1183, y=w1049) -> (x-y=w1186:dbl)
    n618 = Add(x=w1183, y=w1049) -> (x+y=w1187:dbl)
    n619 = Subtract(x=w1078, y=w1060) -> (x-y=w1077:dbl)
    n620 = Subtract(x=w1141, y=w1060) -> (x-y=w1139:dbl)
    n621 = Add(x=w1078, y=w1060) -> (x+y=w1076:dbl)
    n622 = Add(x=w1141, y=w1060) -> (x+y=w1140:dbl)
    n623 = Subtract(x=w1059, y=w1060) -> (x-y=w1061:dbl)
    n624 = Subtract(x=w1188, y=w1060) -> (x-y=w1191:dbl)
    n625 = Add(x=w1059, y=w1060) -> (x+y=w1063:dbl)
    n626 = Add(x=w1188, y=w1060) -> (x+y=w1192:dbl)
    n627 = call-poly <vilib>:"Butterworth Filter.vi"("init/cont (init:F)"=TRUE, "order"=w1014, "filter type"=w1108, "low cutoff freq: fl"=w1114, "high cutoff freq: fh"=w1115, "sampling freq: fs"=w1112, "X"=w1111) -> ("Filtered X"=w1107:cdb[])  [unwired: 1 in, 1 out]
    n628 = call-poly <vilib>:"Butterworth Filter.vi"("init/cont (init:F)"=TRUE, "order"=w1014, "filter type"=w1108, "low cutoff freq: fl"=w1158, "high cutoff freq: fh"=w1159, "sampling freq: fs"=w1112, "X"=w1111) -> ("Filtered X"=w1156:cdb[])  [unwired: 1 in, 1 out]
    n629 = call-poly <vilib>:"Butterworth Filter.vi"("init/cont (init:F)"=TRUE, "order"=w1014, "filter type"=w1108, "low cutoff freq: fl"=w1122, "high cutoff freq: fh"=w1123, "sampling freq: fs"=w1112, "X"=w1111) -> ("Filtered X"=w1120:cdb[])  [unwired: 1 in, 1 out]
    n630 = call-poly <vilib>:"Butterworth Filter.vi"("init/cont (init:F)"=TRUE, "order"=w1014, "filter type"=w1108, "low cutoff freq: fl"=w1200, "high cutoff freq: fh"=w1201, "sampling freq: fs"=w1112, "X"=w1111) -> ("Filtered X"=w1198:cdb[])  [unwired: 1 in, 1 out]
    n631 = call-poly <vilib>:"Butterworth Filter.vi"("init/cont (init:F)"=TRUE, "order"=w1014, "filter type"=w1012, "low cutoff freq: fl"=w1195, "high cutoff freq: fh"=w1196, "sampling freq: fs"=w1092, "X"=w1093) -> ("Filtered X"=w1194:cdb[])  [unwired: 1 in, 1 out]
    n632 = call-poly <vilib>:"Butterworth Filter.vi"("init/cont (init:F)"=TRUE, "order"=w1013, "filter type"=w1042, "low cutoff freq: fl"=w1046, "high cutoff freq: fh"=w1045, "sampling freq: fs"=w1047, "X"=w1048) -> ("Filtered X"=w1043:cdb[])  [unwired: 1 in, 1 out]
    n633 = call-poly <vilib>:"Butterworth Filter.vi"("init/cont (init:F)"=TRUE, "order"=w1014, "filter type"=w1012, "low cutoff freq: fl"=w1098, "high cutoff freq: fh"=w1099, "sampling freq: fs"=w1092, "X"=w1093) -> ("Filtered X"=w1097:cdb[])  [unwired: 1 in, 1 out]
    n634 = call-poly <vilib>:"Butterworth Filter.vi"("init/cont (init:F)"=TRUE, "order"=w1014, "filter type"=w1012, "low cutoff freq: fl"=w1084, "high cutoff freq: fh"=w1083, "sampling freq: fs"=w1092, "X"=w1093) -> ("Filtered X"=w1090:cdb[])  [unwired: 1 in, 1 out]
    n635 = call-poly <vilib>:"Butterworth Filter.vi"("init/cont (init:F)"=TRUE, "order"=w1013, "filter type"=w1042, "low cutoff freq: fl"=w1055, "high cutoff freq: fh"=w1056, "sampling freq: fs"=w1047, "X"=w1048) -> ("Filtered X"=w1058:cdb[])  [unwired: 1 in, 1 out]
    n636 = call-poly <vilib>:"Butterworth Filter.vi"("init/cont (init:F)"=TRUE, "order"=w1014, "filter type"=w1012, "low cutoff freq: fl"=w1148, "high cutoff freq: fh"=w1149, "sampling freq: fs"=w1092, "X"=w1093) -> ("Filtered X"=w1147:cdb[])  [unwired: 1 in, 1 out]
    n637 = call-poly <vilib>:"Butterworth Filter.vi"("init/cont (init:F)"=TRUE, "order"=w1013, "filter type"=w1042, "low cutoff freq: fl"=w1131, "high cutoff freq: fh"=w1132, "sampling freq: fs"=w1047, "X"=w1048) -> ("Filtered X"=w1129:cdb[])  [unwired: 1 in, 1 out]
    n638 = call-poly <vilib>:"Butterworth Filter.vi"("init/cont (init:F)"=TRUE, "order"=w1013, "filter type"=w1042, "low cutoff freq: fl"=w1186, "high cutoff freq: fh"=w1187, "sampling freq: fs"=w1047, "X"=w1048) -> ("Filtered X"=w1185:cdb[])  [unwired: 1 in, 1 out]
    n639 = call-poly <vilib>:"Butterworth Filter.vi"("init/cont (init:F)"=TRUE, "order"=w1013, "filter type"=w1071, "low cutoff freq: fl"=w1077, "high cutoff freq: fh"=w1076, "sampling freq: fs"=w1062, "X"=w1015) -> ("Filtered X"=w1080:cdb[])  [unwired: 1 in, 1 out]
    n640 = call-poly <vilib>:"Butterworth Filter.vi"("init/cont (init:F)"=TRUE, "order"=w1013, "filter type"=w1071, "low cutoff freq: fl"=w1061, "high cutoff freq: fh"=w1063, "sampling freq: fs"=w1062, "X"=w1015) -> ("Filtered X"=w1070:cdb[])  [unwired: 1 in, 1 out]
    n641 = call-poly <vilib>:"Butterworth Filter.vi"("init/cont (init:F)"=TRUE, "order"=w1013, "filter type"=w1071, "low cutoff freq: fl"=w1139, "high cutoff freq: fh"=w1140, "sampling freq: fs"=w1062, "X"=w1015) -> ("Filtered X"=w1138:cdb[])  [unwired: 1 in, 1 out]
    n642 = call-poly <vilib>:"Butterworth Filter.vi"("init/cont (init:F)"=TRUE, "order"=w1013, "filter type"=w1071, "low cutoff freq: fl"=w1191, "high cutoff freq: fh"=w1192, "sampling freq: fs"=w1062, "X"=w1015) -> ("Filtered X"=w1190:cdb[])  [unwired: 1 in, 1 out]
    n643 = Complex To Polar(r * e^(i*theta)=w1107) -> (r=w1106:dbl[], theta=w988:dbl[])
    n644 = Complex To Polar(r * e^(i*theta)=w1120) -> (r=w1118:dbl[], theta=w994:dbl[])
    n645 = Complex To Polar(r * e^(i*theta)=w1156) -> (r=w1155:dbl[], theta=w1000:dbl[])
    n646 = Complex To Polar(r * e^(i*theta)=w1198) -> (r=w1182:dbl[], theta=w1008:dbl[])
    n647 = Complex To Polar(r * e^(i*theta)=w1097) -> (r=w1096:dbl[], theta=w967:dbl[])
    n648 = Complex To Polar(r * e^(i*theta)=w1090) -> (r=w1089:dbl[], theta=w963:dbl[])
    n649 = Complex To Polar(r * e^(i*theta)=w1194) -> (r=w1169:dbl[], theta=w976:dbl[])
    n650 = Complex To Polar(r * e^(i*theta)=w1147) -> (r=w1146:dbl[], theta=w971:dbl[])
    n651 = local read "DownSamplingRatio"() -> (w1087:i32)
    n652 = local read "DownSamplingRatio"() -> (w956:i32)
    n653 = Complex To Polar(r * e^(i*theta)=w1080) -> (r=w1079:dbl[], theta=w946:dbl[])
    n654 = Complex To Polar(r * e^(i*theta)=w1070) -> (r=w1069:dbl[], theta=w939:dbl[])
    n655 = Complex To Polar(r * e^(i*theta)=w1190) -> (r=w1168:dbl[], theta=w931:dbl[])
    n656 = Complex To Polar(r * e^(i*theta)=w1138) -> (r=w1137:dbl[], theta=w924:dbl[])
    n657 = Complex To Polar(r * e^(i*theta)=w1043) -> (r=w1035:dbl[], theta=w909:dbl[])
    n658 = Complex To Polar(r * e^(i*theta)=w1058) -> (r=w1051:dbl[], theta=w920:dbl[])
    n659 = local read "Waveform Size 1"() -> (w973:dbl)
    n660 = Complex To Polar(r * e^(i*theta)=w1185) -> (r=w1167:dbl[], theta=w905:dbl[])
    n661 = Complex To Polar(r * e^(i*theta)=w1129) -> (r=w1128:dbl[], theta=w901:dbl[])
    n662 = local read "DownSamplingRatio"() -> (w1037:i32)
    n663 = local read "DownSamplingRatio"() -> (w896:i32)
    n664 = local read "Waveform Size 1"() -> (w974:dbl)
    n665 = local read "Waveform Size 2"() -> (w1067:dbl)
    n666 = local read "Waveform Size 2"() -> (w1038:dbl)
    n667 = Divide(x=w973, y=w956) -> (x/y=→"Wave size/ DS":dbl)
    n668 = Divide(x=w974, y=w1087) -> (x/y=w1095:dbl)
    n669 = Divide(x=w974, y=w1087) -> (x/y=w1088:dbl)
    n670 = Divide(x=w974, y=w1087) -> (x/y=w1145:dbl)
    n671 = Divide(x=w973, y=w956) -> (x/y=w1105:dbl)
    n672 = Divide(x=w973, y=w956) -> (x/y=w1154:dbl)
    n673 = Divide(x=w973, y=w956) -> (x/y=w1119:dbl)
    n674 = Divide(x=w973, y=w956) -> (x/y=w1181:dbl)
    n675 = Divide(x=w974, y=w1087) -> (x/y=w1170:dbl)
    n676 = Divide(x=w1067, y=w896) -> (x/y=w1073:dbl)
    n677 = Divide(x=w1038, y=w1037) -> (x/y=w1127:dbl)
    n678 = Divide(x=w1067, y=w896) -> (x/y=w1068:dbl)
    n679 = Divide(x=w1067, y=w896) -> (x/y=w1136:dbl)
    n680 = Divide(x=w1038, y=w1037) -> (x/y=w1036:dbl)
    n681 = Reshape Array(w1096, w1095, w1087) -> (w1101:dbl[][])
    n682 = Divide(x=w1067, y=w896) -> (x/y=w1176:dbl)
    n683 = Reshape Array(w1089, w1088, w1087) -> (w1072:dbl[][])
    n684 = Divide(x=w1038, y=w1037) -> (x/y=w1052:dbl)
    n685 = Divide(x=w1038, y=w1037) -> (x/y=w1173:dbl)
    n686 = Reshape Array(w1146, w1145, w1087) -> (w1144:dbl[][])
    n687 = Reshape Array(w1106, w1105, w956) -> (w1104:dbl[][])
    n688 = Reshape Array(w1118, w1119, w956) -> (w1117:dbl[][])
    n689 = Reshape Array(w1182, w1181, w956) -> (w1180:dbl[][])
    n690 = Reshape Array(w1169, w1170, w1087) -> (w1178:dbl[][])
    n691 = Reshape Array(w1155, w1154, w956) -> (w1153:dbl[][])
    n692 = Reshape Array(w1079, w1073, w896) -> (w1075:dbl[][])
    n693 = Reshape Array(w1128, w1127, w1037) -> (w1126:dbl[][])
    n694 = Reshape Array(w1069, w1068, w896) -> (w1066:dbl[][])
    n695 = Reshape Array(w1137, w1136, w896) -> (w1135:dbl[][])
    n696 = Reshape Array(w1035, w1036, w1037) -> (w1040:dbl[][])
    n697 = Reshape Array(w1168, w1176, w896) -> (w1175:dbl[][])
    n698 = Reshape Array(w1051, w1052, w1037) -> (w1053:dbl[][])
    n699 = Reshape Array(w1167, w1173, w1037) -> (w1172:dbl[][])
    n700 = for {
      tunnel: w1180 -> [w1283] mode=indexing
      tunnel: [w1282] -> w1179 mode=indexing
      workers-P: _ -> [_]
      n701 = Add Array Elements(numeric array=w1283) -> (sum=w1282:dbl)
    }
    n702 = for {
      tunnel: w1153 -> [w1268] mode=indexing
      tunnel: [w1267] -> w1152 mode=indexing
      workers-P: _ -> [_]
      n703 = Add Array Elements(numeric array=w1268) -> (sum=w1267:dbl)
    }
    n704 = for {
      tunnel: w1117 -> [w1260] mode=indexing
      tunnel: [w1259] -> w1116 mode=indexing
      workers-P: _ -> [_]
      n705 = Add Array Elements(numeric array=w1260) -> (sum=w1259:dbl)
    }
    n706 = for {
      tunnel: w1104 -> [w1258] mode=indexing
      tunnel: [w1257] -> w1103 mode=indexing
      workers-P: _ -> [_]
      n707 = Add Array Elements(numeric array=w1258) -> (sum=w1257:dbl)
    }
    n708 = for {
      tunnel: w1101 -> [w1256] mode=indexing
      tunnel: [w1255] -> w1102 mode=indexing
      workers-P: _ -> [_]
      n709 = Add Array Elements(numeric array=w1256) -> (sum=w1255:dbl)
    }
    n710 = for {
      tunnel: w1178 -> [w1281] mode=indexing
      tunnel: [w1280] -> w1177 mode=indexing
      workers-P: _ -> [_]
      n711 = Add Array Elements(numeric array=w1281) -> (sum=w1280:dbl)
    }
    n712 = for {
      tunnel: w1072 -> [w1254] mode=indexing
      tunnel: [w1253] -> w1086 mode=indexing
      workers-P: _ -> [_]
      n713 = Add Array Elements(numeric array=w1254) -> (sum=w1253:dbl)
    }
    n714 = for {
      tunnel: w1144 -> [w1266] mode=indexing
      tunnel: [w1265] -> w1143 mode=indexing
      workers-P: _ -> [_]
      n715 = Add Array Elements(numeric array=w1266) -> (sum=w1265:dbl)
    }
    n716 = for {
      tunnel: w1075 -> [w1252] mode=indexing
      tunnel: [w1251] -> w1074 mode=indexing
      workers-P: _ -> [_]
      n717 = Add Array Elements(numeric array=w1252) -> (sum=w1251:dbl)
    }
    n718 = for {
      tunnel: w1066 -> [w1250] mode=indexing
      tunnel: [w1249] -> w1065 mode=indexing
      workers-P: _ -> [_]
      n719 = Add Array Elements(numeric array=w1250) -> (sum=w1249:dbl)
    }
    n720 = for {
      tunnel: w1135 -> [w1264] mode=indexing
      tunnel: [w1263] -> w1134 mode=indexing
      workers-P: _ -> [_]
      n721 = Add Array Elements(numeric array=w1264) -> (sum=w1263:dbl)
    }
    n722 = for {
      tunnel: w1040 -> [w1246] mode=indexing
      tunnel: [w1245] -> w1039 mode=indexing
      workers-P: _ -> [_]
      n723 = Add Array Elements(numeric array=w1246) -> (sum=w1245:dbl)
    }
    n724 = for {
      tunnel: w1175 -> [w1279] mode=indexing
      tunnel: [w1278] -> w1174 mode=indexing
      workers-P: _ -> [_]
      n725 = Add Array Elements(numeric array=w1279) -> (sum=w1278:dbl)
    }
    n726 = for {
      tunnel: w1053 -> [w1248] mode=indexing
      tunnel: [w1247] -> w1050 mode=indexing
      workers-P: _ -> [_]
      n727 = Add Array Elements(numeric array=w1248) -> (sum=w1247:dbl)
    }
    n728 = for {
      tunnel: w1172 -> [w1277] mode=indexing
      tunnel: [w1276] -> w1171 mode=indexing
      workers-P: _ -> [_]
      n729 = Add Array Elements(numeric array=w1277) -> (sum=w1276:dbl)
    }
    n730 = for {
      tunnel: w1126 -> [w1262] mode=indexing
      tunnel: [w1261] -> w1125 mode=indexing
      workers-P: _ -> [_]
      n731 = Add Array Elements(numeric array=w1262) -> (sum=w1261:dbl)
    }
    n732 = Divide(x=w1102, y=w1087) -> (x/y=w1029:dbl[])
    n733 = Divide(x=w1086, y=w1087) -> (x/y=w1028:dbl[])
    n734 = Divide(x=w1143, y=w1087) -> (x/y=w1030:dbl[])
    n735 = Divide(x=w1179, y=w956) -> (x/y=w1166:dbl[])
    n736 = Divide(x=w1177, y=w1087) -> (x/y=w1031:dbl[])
    n737 = Divide(x=w1152, y=w956) -> (x/y=w1034:dbl[])
    n738 = Divide(x=w1116, y=w956) -> (x/y=w1033:dbl[])
    n739 = Divide(x=w1103, y=w956) -> (x/y=w1032:dbl[])
    n740 = Divide(x=w1074, y=w896) -> (x/y=w1027:dbl[])
    n741 = Divide(x=w1065, y=w896) -> (x/y=w1026:dbl[])
    n742 = Divide(x=w1174, y=w896) -> (x/y=w1025:dbl[])
    n743 = Divide(x=w1134, y=w896) -> (x/y=w1024:dbl[])
    n744 = Divide(x=w1039, y=w1037) -> (x/y=w1021:dbl[])
    n745 = Divide(x=w1171, y=w1037) -> (x/y=w1022:dbl[])
    n746 = Divide(x=w1050, y=w1037) -> (x/y=w1020:dbl[])
    n747 = Divide(x=w1125, y=w1037) -> (x/y=w1023:dbl[])
    n748 = local read "Tx ch3  ph"() -> (w993:cdb[])
    n749 = local read "Tx ch3  ph"() -> (w966:cdb[])
    n750 = local read "Acq Started"() -> (w1016:bool)
    n751 = local read "Tx ch1  ph"() -> (w1007:cdb[])
    n752 = local read "Tx ch2  ph"() -> (w1001:cdb[])
    n753 = local read "Tx ch2  ph"() -> (w970:cdb[])
    n754 = Subtract(x=w971, y=w970) -> (x-y=w969:cdb[])
    n755 = local read "Tx ch1  ph"() -> (w975:cdb[])
    n756 = local read "Tx ch4 ph"() -> (w962:cdb[])
    n757 = Subtract(x=w1000, y=w1001) -> (x-y=w999:cdb[])
    n758 = Subtract(x=w967, y=w966) -> (x-y=w965:cdb[])
    n759 = Subtract(x=w963, y=w962) -> (x-y=w961:cdb[])
    n760 = call <vilib>:"Unwrap Phase.vi"("phase unit"=w960, "Phase"=w969) -> ("Unwrapped Phase"=w979:dbl[])  [unwired: 8 in, 1 out]
    n761 = Subtract(x=w976, y=w975) -> (x-y=w982:cdb[])
    n762 = local read "Tx ch4 ph"() -> (w987:cdb[])
    n763 = local read "Buffer"() -> (w1017:bool)
    n764 = Subtract(x=w988, y=w987) -> (x-y=w986:cdb[])
    n765 = local read "Wave size/ DS"() -> (w958:dbl)
    n766 = local read "Flush"() -> (w1161:bool)
    n767 = call <vilib>:"Unwrap Phase.vi"("phase unit"=w960, "Phase"=w961) -> ("Unwrapped Phase"=w959:dbl[])  [unwired: 8 in, 1 out]
    n768 = call <vilib>:"Unwrap Phase.vi"("phase unit"=w960, "Phase"=w965) -> ("Unwrapped Phase"=w968:dbl[])  [unwired: 8 in, 1 out]
    n769 = call <vilib>:"Unwrap Phase.vi"("phase unit"=w960, "Phase"=w982) -> ("Unwrapped Phase"=w983:dbl[])  [unwired: 8 in, 1 out]
    n770 = call <vilib>:"Unwrap Phase.vi"("phase unit"=w960, "Phase"=w999) -> ("Unwrapped Phase"=w998:dbl[])  [unwired: 8 in, 1 out]
    n771 = Subtract(x=w1008, y=w1007) -> (x-y=w1006:cdb[])
    n772 = Subtract(x=w994, y=w993) -> (x-y=w992:cdb[])
    n773 = call <vilib>:"Unwrap Phase.vi"("phase unit"=w960, "Phase"=w992) -> ("Unwrapped Phase"=w995:dbl[])  [unwired: 8 in, 1 out]
    n774 = call <vilib>:"Unwrap Phase.vi"("phase unit"=w960, "Phase"=w986) -> ("Unwrapped Phase"=w989:dbl[])  [unwired: 8 in, 1 out]
    n775 = And(x=w1016, y=w1017) -> (x .and. y?=w1018:bool)
    n776 = local read "Tx ch3  ph"() -> (w930:cdb[])
    n777 = call <vilib>:"Unwrap Phase.vi"("phase unit"=w960, "Phase"=w1006) -> ("Unwrapped Phase"=w1003:dbl[])  [unwired: 8 in, 1 out]
    n778 = local read "Tx ch2  ph"() -> (w910:cdb[])
    n779 = local read "Tx ch4 ph"() -> (w925:cdb[])
    n780 = Reshape Array(w979, w958, w956) -> (w981:dbl[][])
    n781 = Divide(x=w973, y=w956) -> (x/y=w1002:dbl)
    n782 = Divide(x=w973, y=w956) -> (x/y=w1011:dbl)
    n783 = Reshape Array(w968, w958, w956) -> (w978:dbl[][])
    n784 = Reshape Array(w959, w958, w956) -> (w957:dbl[][])
    n785 = local read "Tx ch3  ph"() -> (w906:cdb[])
    n786 = local read "Tx ch4 ph"() -> (w902:cdb[])
    n787 = Reshape Array(w983, w958, w956) -> (w985:dbl[][])
    n788 = local read "Tx ch2  ph"() -> (w938:cdb[])
    n789 = local read "Tx ch1  ph"() -> (w919:cdb[])
    n790 = Reshape Array(w989, w958, w956) -> (w991:dbl[][])
    n791 = Reshape Array(w995, w958, w956) -> (w997:dbl[][])
    n792 = Reshape Array(w998, w1002, w956) -> (w1005:dbl[][])
    n793 = Reshape Array(w1003, w1011, w956) -> (w1010:dbl[][])
    n794 = for {
      tunnel: w981 -> [w1234] mode=indexing
      tunnel: [w1233] -> w980 mode=indexing
      workers-P: _ -> [_]
      n795 = Add Array Elements(numeric array=w1234) -> (sum=w1233:dbl)
    }
    n796 = for {
      tunnel: w978 -> [w1232] mode=indexing
      tunnel: [w1231] -> w977 mode=indexing
      workers-P: _ -> [_]
      n797 = Add Array Elements(numeric array=w1232) -> (sum=w1231:dbl)
    }
    n798 = for {
      tunnel: w957 -> [w1230] mode=indexing
      tunnel: [w1229] -> w964 mode=indexing
      workers-P: _ -> [_]
      n799 = Add Array Elements(numeric array=w1230) -> (sum=w1229:dbl)
    }
    n800 = for {
      tunnel: w985 -> [w1236] mode=indexing
      tunnel: [w1235] -> w984 mode=indexing
      workers-P: _ -> [_]
      n801 = Add Array Elements(numeric array=w1236) -> (sum=w1235:dbl)
    }
    n802 = Subtract(x=w931, y=w930) -> (x-y=w929:cdb[])
    n803 = for {
      tunnel: w991 -> [w1238] mode=indexing
      tunnel: [w1237] -> w990 mode=indexing
      workers-P: _ -> [_]
      n804 = Add Array Elements(numeric array=w1238) -> (sum=w1237:dbl)
    }
    n805 = Subtract(x=w924, y=w925) -> (x-y=w923:cdb[])
    n806 = Subtract(x=w920, y=w919) -> (x-y=w918:cdb[])
    n807 = Subtract(x=w909, y=w910) -> (x-y=w908:cdb[])
    n808 = Subtract(x=w905, y=w906) -> (x-y=w904:cdb[])
    n809 = for {
      tunnel: w997 -> [w1240] mode=indexing
      tunnel: [w1239] -> w996 mode=indexing
      workers-P: _ -> [_]
      n810 = Add Array Elements(numeric array=w1240) -> (sum=w1239:dbl)
    }
    n811 = Subtract(x=w901, y=w902) -> (x-y=w900:cdb[])
    n812 = for {
      tunnel: w1005 -> [w1242] mode=indexing
      tunnel: [w1241] -> w1004 mode=indexing
      workers-P: _ -> [_]
      n813 = Add Array Elements(numeric array=w1242) -> (sum=w1241:dbl)
    }
    n814 = for {
      tunnel: w1010 -> [w1244] mode=indexing
      tunnel: [w1243] -> w1009 mode=indexing
      workers-P: _ -> [_]
      n815 = Add Array Elements(numeric array=w1244) -> (sum=w1243:dbl)
    }
    n816 = local read "Wave size/ DS"() -> (w897:dbl)
    n817 = Subtract(x=w939, y=w938) -> (x-y=w937:cdb[])
    n818 = call <vilib>:"Unwrap Phase.vi"("phase unit"=w899, "Phase"=w929) -> ("Unwrapped Phase"=w928:dbl[])  [unwired: 8 in, 1 out]
    n819 = call <vilib>:"Unwrap Phase.vi"("phase unit"=w899, "Phase"=w918) -> ("Unwrapped Phase"=w917:dbl[])  [unwired: 8 in, 1 out]
    n820 = call <vilib>:"Unwrap Phase.vi"("phase unit"=w899, "Phase"=w908) -> ("Unwrapped Phase"=w907:dbl[])  [unwired: 8 in, 1 out]
    n821 = call <vilib>:"Unwrap Phase.vi"("phase unit"=w899, "Phase"=w904) -> ("Unwrapped Phase"=w903:dbl[])  [unwired: 8 in, 1 out]
    n822 = call <vilib>:"Unwrap Phase.vi"("phase unit"=w899, "Phase"=w900) -> ("Unwrapped Phase"=w898:dbl[])  [unwired: 8 in, 1 out]
    n823 = call <vilib>:"Unwrap Phase.vi"("phase unit"=w899, "Phase"=w923) -> ("Unwrapped Phase"=w926:dbl[])  [unwired: 8 in, 1 out]
    n824 = local read "Wave size/ DS"() -> (w927:dbl)
    n825 = local read "Tx ch1  ph"() -> (w945:cdb[])
    n826 = call <vilib>:"Unwrap Phase.vi"("phase unit"=w899, "Phase"=w937) -> ("Unwrapped Phase"=w936:dbl[])  [unwired: 8 in, 1 out]
    n827 = Subtract(x=w946, y=w945) -> (x-y=w944:cdb[])
    n828 = call <vilib>:"Unwrap Phase.vi"("phase unit"=w899, "Phase"=w944) -> ("Unwrapped Phase"=w943:dbl[])  [unwired: 8 in, 1 out]
    n829 = Divide(x=w990, y=w956) -> (x/y=w951:dbl[])
    n830 = Reshape Array(w928, w897, w896) -> (w934:dbl[][])
    n831 = Divide(x=w977, y=w956) -> (x/y=w948:dbl[])
    n832 = Divide(x=w964, y=w956) -> (x/y=w947:dbl[])
    n833 = Reshape Array(w917, w897, w896) -> (w921:dbl[][])
    n834 = Divide(x=w984, y=w956) -> (x/y=w950:dbl[])
    n835 = Divide(x=w980, y=w956) -> (x/y=w949:dbl[])
    n836 = Divide(x=w996, y=w956) -> (x/y=w952:dbl[])
    n837 = Reshape Array(w907, w897, w896) -> (w915:dbl[][])
    n838 = Reshape Array(w903, w897, w896) -> (w913:dbl[][])
    n839 = Divide(x=w1004, y=w956) -> (x/y=w953:dbl[])
    n840 = Reshape Array(w898, w897, w896) -> (w911:dbl[][])
    n841 = Reshape Array(w926, w897, w896) -> (w932:dbl[][])
    n842 = Divide(x=w1009, y=w956) -> (x/y=w954:dbl[])
    n843 = Reshape Array(w936, w897, w896) -> (w940:dbl[][])
    n844 = Reshape Array(w943, w927, w896) -> (w942:dbl[][])
    n845 = for {
      tunnel: w934 -> [w1224] mode=indexing
      tunnel: [w1223] -> w935 mode=indexing
      workers-P: _ -> [_]
      n846 = Add Array Elements(numeric array=w1224) -> (sum=w1223:dbl)
    }
    n847 = for {
      tunnel: w921 -> [w1220] mode=indexing
      tunnel: [w1219] -> w922 mode=indexing
      workers-P: _ -> [_]
      n848 = Add Array Elements(numeric array=w1220) -> (sum=w1219:dbl)
    }
    n849 = for {
      tunnel: w915 -> [w1218] mode=indexing
      tunnel: [w1217] -> w916 mode=indexing
      workers-P: _ -> [_]
      n850 = Add Array Elements(numeric array=w1218) -> (sum=w1217:dbl)
    }
    n851 = for {
      tunnel: w913 -> [w1216] mode=indexing
      tunnel: [w1215] -> w914 mode=indexing
      workers-P: _ -> [_]
      n852 = Add Array Elements(numeric array=w1216) -> (sum=w1215:dbl)
    }
    n853 = for {
      tunnel: w911 -> [w1214] mode=indexing
      tunnel: [w1213] -> w912 mode=indexing
      workers-P: _ -> [_]
      n854 = Add Array Elements(numeric array=w1214) -> (sum=w1213:dbl)
    }
    n855 = for {
      tunnel: w932 -> [w1222] mode=indexing
      tunnel: [w1221] -> w933 mode=indexing
      workers-P: _ -> [_]
      n856 = Add Array Elements(numeric array=w1222) -> (sum=w1221:dbl)
    }
    n857 = for {
      tunnel: w940 -> [w1226] mode=indexing
      tunnel: [w1225] -> w941 mode=indexing
      workers-P: _ -> [_]
      n858 = Add Array Elements(numeric array=w1226) -> (sum=w1225:dbl)
    }
    n859 = for {
      tunnel: w942 -> [w1228] mode=indexing
      tunnel: [w1227] -> w955 mode=indexing
      workers-P: _ -> [_]
      n860 = Add Array Elements(numeric array=w1228) -> (sum=w1227:dbl)
    }
    n861 = Divide(x=w935, y=w896) -> (x/y=w893:dbl[])
    n862 = Divide(x=w922, y=w896) -> (x/y=w891:dbl[])
    n863 = Divide(x=w916, y=w896) -> (x/y=w890:dbl[])
    n864 = Divide(x=w914, y=w896) -> (x/y=w889:dbl[])
    n865 = Divide(x=w912, y=w896) -> (x/y=w888:dbl[])
    n866 = Divide(x=w933, y=w896) -> (x/y=w892:dbl[])
    n867 = Divide(x=w941, y=w896) -> (x/y=w894:dbl[])
    n868 = Divide(x=w955, y=w896) -> (x/y=w895:dbl[])
    n869 = Build Array(w1166, w954, w1034, w953, w1033, w952, w1032, w951, w1031, w950, w1030, w949, w1029, w948, w1028, w947, w1027, w895, w1026, w894, w1025, w893, w1024, w892, w1020, w891, w1021, w890, w1022, w889, w1023, w888) -> (w1164:dbl[][])
    "ChAmp" <- w1164
    n870 = case shown="True" w1018 {
      tunnel: w1163 -> [w1271 w1275]
      tunnel: w1164 -> [_ w1274]
      tunnel: w1161 -> [w1270 _]
      tunnel: w1019 -> [w1269 _]
      frame False {
        n871 = case shown="True" w1270 {
          tunnel: w1271 -> [_ w1273]
          tunnel: w1269 -> [_ w1272]
          frame False {
          }
          frame True {
            n872 = Flush Queue(queue=w1272) -> ()  [unwired: 1 in, 3 out]
            n873 = Flush Queue(queue=w1273) -> ()  [unwired: 1 in, 3 out]
          }
        }
      }
      frame True {
        n874 = Enqueue Element(queue=w1275, element=w1274) -> ()  [unwired: 2 in, 3 out]
      }
    }
    n875 = Enqueue Element(queue=w1165, element=w1164) -> ()  [unwired: 2 in, 3 out]
  }
  n876 = local read "DownSamplingRatio"() -> (w50:i32)
  n877 = local read "Waveform Size 1"() -> (w51:dbl)
  n878 = Divide(x=w51, y=w50) -> (x/y=w37:dbl)
  n879 = Divide(x=w37, y="DownSamplingRatio 2") -> (x/y=w28:dbl)
  n880 = Multiply(x=w27, y=w28) -> (x*y=w45:dbl)
  n881 = Initialize Array(w26, w27, w28) -> (w49:dbl[][])
  n882 = Initialize Array(w26, w27, w28) -> (w48:dbl[][])
  n883 = Initialize Array(w26, w27, w28) -> (w47:dbl[][])
  n884 = Initialize Array(w26, w27, w28) -> (w46:dbl[][])
  n885 = Initialize Array(w26, w27, w28) -> (w25:dbl[][])
  n886 = Initialize Array(w26, w27, w28) -> (w24:dbl[][])
  n887 = Initialize Array(w26, w27, w28) -> (w23:dbl[][])
  n888 = Initialize Array(w26, w27, w28) -> (w22:dbl[][])
  n889 = while {
    tunnel: w27 -> [w1397]
    tunnel: w52 -> [w1390]
    shift-right: [w1387] -> _
    shift-left: w49 -> [w1369]
    tunnel: w45 -> [w1305]
    shift-right: [w1381] -> _
    shift-left: w48 -> [w1393]
    shift-right: [w1380] -> _
    shift-left: w47 -> [w1392]
    shift-right: [w1379] -> _
    shift-left: w46 -> [w1391]
    tunnel: "DownSamplingRatio 2" -> [w1320]
    tunnel: w28 -> [w1329]
    tunnel: "DownSamplingRatio 2" -> [w1353]
    shift-right: [w1301] -> _
    shift-left: w25 -> [w1315]
    shift-right: [w1300] -> _
    shift-left: w24 -> [w1307]
    shift-right: [w1299] -> _
    shift-left: w23 -> [w1310]
    shift-right: [w1298] -> _
    shift-left: w22 -> [w1317]
    stop <- FALSE stop-if-true
    # "Tx4 to Rx4 QueInd_15"
    # "Tx3 to Rx4 QueInd_14"
    # "Tx2 to Rx4 QueInd_13"
    # "Tx1 to Rx4 QueInd_12"
    # "Tx4 to Rx3 QueInd_11"
    # "Tx3 to Rx3 QueInd_10"
    # "Tx2 to Rx3 QueInd_9"
    # "Tx1 to Rx3 QueInd_8"
    # "Tx4 to Rx2 QueInd_7"
    # "Tx3 to Rx2 QueInd_6"
    # "Tx2 to Rx2 QueInd_5"
    # "Tx1 to Rx2 QueInd_4"
    # "Tx4 to Rx1 QueInd_3"
    # "Tx3 to Rx1 QueInd_2"
    # "Tx2 to Rx1 QueInd_1"
    # "Tx1 to Rx1 QueInd_0"
    n890 = local read "Sampling Rate"() -> (w1354:dbl)
    n891 = Get Queue Status(queue=w1390) -> (# elements in queue=→"# elements in view queue":i32)  [unwired: 2 in, 7 out]
    n892 = Dequeue Element(queue=w1390) -> (element=w1334:dbl[][])  [unwired: 2 in, 3 out]
    n893 = Decrement(x=w1397) -> (x-1=w1308:i32)
    n894 = Divide(x=w1354, y=w1353) -> (x/y=→"Dis Sampling Rate":dbl)
    n895 = Index Array(array=w1334, index (row)=10 ("index")) -> (element=w1333:dbl[])  [unwired: 1 in]
    n896 = Index Array(array=w1334, index (row)=11 ("index")) -> (element=w1332:dbl[])  [unwired: 1 in]
    n897 = Index Array(array=w1334, index (row)=15 ("index")) -> (element=w1331:dbl[])  [unwired: 1 in]
    n898 = Index Array(array=w1334, index (row)=14 ("index")) -> (element=w1330:dbl[])  [unwired: 1 in]
    n899 = Index Array(array=w1334, index (row)=0 ("index")) -> (element=w1367:dbl[])  [unwired: 1 in]
    n900 = Index Array(array=w1334, index (row)=1 ("index")) -> (element=w1366:dbl[])  [unwired: 1 in]
    n901 = Index Array(array=w1334, index (row)=5 ("index")) -> (element=w1365:dbl[])  [unwired: 1 in]
    n902 = Index Array(array=w1334, index (row)=4 ("index")) -> (element=w1364:dbl[])  [unwired: 1 in]
    n903 = Array Subset(array=w1310, index (row)=0 ("index"), length (row)=w1308) -> (w1309:dbl[][])  [unwired: 2 in]
    n904 = Array Subset(array=w1317, index (row)=0 ("index"), length (row)=w1308) -> (w1316:dbl[][])  [unwired: 2 in]
    n905 = Array Subset(array=w1307, index (row)=0 ("index"), length (row)=w1308) -> (w1306:dbl[][])  [unwired: 2 in]
    n906 = Array Subset(array=w1315, index (row)=0 ("index"), length (row)=w1308) -> (w1314:dbl[][])  [unwired: 2 in]
    n907 = Array Subset(array=w1369, index (row)=0 ("index"), length (row)=w1308) -> (w1388:dbl[][])  [unwired: 2 in]
    n908 = Array Subset(array=w1393, index (row)=0 ("index"), length (row)=w1308) -> (w1384:dbl[][])  [unwired: 2 in]
    n909 = Array Subset(array=w1392, index (row)=0 ("index"), length (row)=w1308) -> (w1383:dbl[][])  [unwired: 2 in]
    n910 = Array Subset(array=w1391, index (row)=0 ("index"), length (row)=w1308) -> (w1382:dbl[][])  [unwired: 2 in]
    n911 = Reshape Array(w1332, w1329, w1320) -> (w1327:dbl[][])
    n912 = Reshape Array(w1331, w1329, w1320) -> (w1326:dbl[][])
    n913 = Reshape Array(w1330, w1329, w1320) -> (w1325:dbl[][])
    n914 = Reshape Array(w1366, w1329, w1320) -> (w1361:dbl[][])
    n915 = Reshape Array(w1365, w1329, w1320) -> (w1360:dbl[][])
    n916 = Reshape Array(w1364, w1329, w1320) -> (w1359:dbl[][])
    n917 = Reshape Array(w1333, w1329, w1320) -> (w1328:dbl[][])
    n918 = Reshape Array(w1367, w1329, w1320) -> (w1363:dbl[][])
    n919 = for {
      tunnel: w1326 -> [w1407] mode=indexing
      tunnel: [w1406] -> w1322 mode=indexing
      workers-P: _ -> [_]
      n920 = Add Array Elements(numeric array=w1407) -> (sum=w1406:dbl)
    }
    n921 = for {
      tunnel: w1325 -> [w1405] mode=indexing
      tunnel: [w1404] -> w1321 mode=indexing
      workers-P: _ -> [_]
      n922 = Add Array Elements(numeric array=w1405) -> (sum=w1404:dbl)
    }
    n923 = for {
      tunnel: w1360 -> [w1415] mode=indexing
      tunnel: [w1414] -> w1357 mode=indexing
      workers-P: _ -> [_]
      n924 = Add Array Elements(numeric array=w1415) -> (sum=w1414:dbl)
    }
    n925 = for {
      tunnel: w1359 -> [w1413] mode=indexing
      tunnel: [w1412] -> w1356 mode=indexing
      workers-P: _ -> [_]
      n926 = Add Array Elements(numeric array=w1413) -> (sum=w1412:dbl)
    }
    n927 = for {
      tunnel: w1327 -> [w1409] mode=indexing
      tunnel: [w1408] -> w1323 mode=indexing
      workers-P: _ -> [_]
      n928 = Add Array Elements(numeric array=w1409) -> (sum=w1408:dbl)
    }
    n929 = for {
      tunnel: w1361 -> [w1417] mode=indexing
      tunnel: [w1416] -> w1358 mode=indexing
      workers-P: _ -> [_]
      n930 = Add Array Elements(numeric array=w1417) -> (sum=w1416:dbl)
    }
    n931 = for {
      tunnel: w1328 -> [w1411] mode=indexing
      tunnel: [w1410] -> w1324 mode=indexing
      workers-P: _ -> [_]
      n932 = Add Array Elements(numeric array=w1411) -> (sum=w1410:dbl)
    }
    n933 = for {
      tunnel: w1363 -> [w1419] mode=indexing
      tunnel: [w1418] -> w1362 mode=indexing
      workers-P: _ -> [_]
      n934 = Add Array Elements(numeric array=w1419) -> (sum=w1418:dbl)
    }
    n935 = Divide(x=w1324, y=w1320) -> (x/y=w1289:dbl[])
    n936 = Divide(x=w1362, y=w1320) -> (x/y=w1291:dbl[])
    n937 = Divide(x=w1323, y=w1320) -> ()  [unwired: 1 out]
    n938 = Divide(x=w1322, y=w1320) -> (x/y=w1288:dbl[])
    n939 = Divide(x=w1358, y=w1320) -> ()  [unwired: 1 out]
    n940 = Divide(x=w1357, y=w1320) -> (x/y=w1290:dbl[])
    n941 = Divide(x=w1321, y=w1320) -> ()  [unwired: 1 out]
    n942 = Divide(x=w1356, y=w1320) -> ()  [unwired: 1 out]
    n943 = Build Array (concatenate)(w1288, w1309) -> (w1299:dbl[][])
    n944 = Build Array (concatenate)(w1288, w1316) -> (w1298:dbl[][])
    n945 = Build Array (concatenate)(w1289, w1306) -> (w1300:dbl[][])
    n946 = Build Array (concatenate)(w1289, w1314) -> (w1301:dbl[][])
    n947 = Build Array (concatenate)(w1290, w1382) -> (w1379:dbl[][])
    n948 = Build Array (concatenate)(w1290, w1383) -> (w1380:dbl[][])
    n949 = Build Array (concatenate)(w1291, w1384) -> (w1381:dbl[][])
    n950 = Build Array (concatenate)(w1291, w1388) -> (w1387:dbl[][])
    n951 = Reshape Array(w1299, w1305) -> (w1303:dbl[])
    n952 = Reshape Array(w1298, w1305) -> (w1302:dbl[])
    n953 = Reshape Array(w1300, w1305) -> (w1304:dbl[])
    n954 = Reshape Array(w1301, w1305) -> (w1313:dbl[])
    n955 = Reshape Array(w1379, w1305) -> (w1340:dbl[])
    n956 = Reshape Array(w1380, w1305) -> (w1341:dbl[])
    n957 = Reshape Array(w1381, w1305) -> (w1342:dbl[])
    n958 = Reshape Array(w1387, w1305) -> (w1343:dbl[])
    n959 = local read "Dis Sampling Rate"() -> (w1344:dbl)
    n960 = call-poly <vilib>:"Butterworth Filter.vi"("init/cont (init:F)"=TRUE, "order"=3, "filter type"="top filter", "low cutoff freq: fl"="fl Top", "high cutoff freq: fh"="fh Top", "sampling freq: fs"=w1344, "X"=w1343) -> ("Filtered X"=w1339:dbl[])  [unwired: 1 in, 1 out]
    n961 = call-poly <vilib>:"Butterworth Filter.vi"("init/cont (init:F)"=TRUE, "order"=3, "filter type"="bottom filter", "low cutoff freq: fl"="fl Bottom", "high cutoff freq: fh"="fh Bottom", "sampling freq: fs"=w1344, "X"=w1342) -> ("Filtered X"=w1372:dbl[])  [unwired: 1 in, 1 out]
    n962 = call-poly <vilib>:"Butterworth Filter.vi"("init/cont (init:F)"=TRUE, "order"=3, "filter type"="top filter", "low cutoff freq: fl"="fl Top", "high cutoff freq: fh"="fh Top", "sampling freq: fs"=w1344, "X"=w1313) -> ("Filtered X"=w1297:dbl[])  [unwired: 1 in, 1 out]
    n963 = call-poly <vilib>:"Butterworth Filter.vi"("init/cont (init:F)"=TRUE, "order"=3, "filter type"="bottom filter", "low cutoff freq: fl"="fl Bottom", "high cutoff freq: fh"="fh Bottom", "sampling freq: fs"=w1344, "X"=w1304) -> ("Filtered X"=w1296:dbl[])  [unwired: 1 in, 1 out]
    n964 = call-poly <vilib>:"Butterworth Filter.vi"("init/cont (init:F)"=TRUE, "order"=3, "filter type"="top filter", "low cutoff freq: fl"="fl Top", "high cutoff freq: fh"="fh Top", "sampling freq: fs"=w1344, "X"=w1341) -> ("Filtered X"=w1370:dbl[])  [unwired: 1 in, 1 out]
    n965 = call-poly <vilib>:"Butterworth Filter.vi"("init/cont (init:F)"=TRUE, "order"=3, "filter type"="top filter", "low cutoff freq: fl"="fl Top", "high cutoff freq: fh"="fh Top", "sampling freq: fs"=w1344, "X"=w1303) -> ("Filtered X"=w1295:dbl[])  [unwired: 1 in, 1 out]
    n966 = call-poly <vilib>:"Butterworth Filter.vi"("init/cont (init:F)"=TRUE, "order"=3, "filter type"="bottom filter", "low cutoff freq: fl"="fl Bottom", "high cutoff freq: fh"="fh Bottom", "sampling freq: fs"=w1344, "X"=w1340) -> ("Filtered X"=w1371:dbl[])  [unwired: 1 in, 1 out]
    n967 = call-poly <vilib>:"Butterworth Filter.vi"("init/cont (init:F)"=TRUE, "order"=3, "filter type"="bottom filter", "low cutoff freq: fl"="fl Bottom", "high cutoff freq: fh"="fh Bottom", "sampling freq: fs"=w1344, "X"=w1302) -> ("Filtered X"=w1294:dbl[])  [unwired: 1 in, 1 out]
    n968 = Build Array(w1339, w1372, w1370, w1371, w1297, w1296, w1295, w1294) -> (→"8 Ch Heart":dbl[][])
  }
  n969 = while {
    tunnel: w41 -> [w1427]
    tunnel: w32 -> [w1426]
    tunnel: w2 -> [w1422]
    tunnel: [w1420] -> _
    stop <- FALSE stop-if-true
    n970 = Wait (ms)(milliseconds to wait=u32 100) -> ()  [unwired: 1 out]
    n971 = Get Queue Status(queue=w1427) -> (queue out=w1429:refnum<queue>, # elements in queue=w1430:i32)  [unwired: 2 in, 6 out]
    "# NCS Buffer" <- w1430
    n972 = Get Queue Status(queue=w1422) -> (queue out=w1423:refnum<queue>, # elements in queue=w1421:i32)  [unwired: 2 in, 6 out]
    n973 = local read "Save"() -> (w1424:bool)
    n974 = case shown="True" w1424 {
      tunnel: w1430 -> [_ w1500]
      tunnel: w1429 -> [_ w1501]
      tunnel: w1426 -> [_ w1499]
      tunnel: w1423 -> [_ w1440]
      tunnel: w1421 -> [_ w1435]
      tunnel: [_ w1431] -> w1420
      frame False {
      }
      frame True {
        # "Once Saved: Stop saving"
        # "Getting channels from Buffer Queue"
        n975 = Multiply(x=w1500, y=w1499) -> (x*y=w1456:dbl)
        n976 = for {
          N: w1500 -> [_]
          tunnel: [w1710] -> w1472 mode=indexing
          tunnel: [w1706] -> w1471 mode=indexing
          tunnel: [w1705] -> w1469 mode=indexing
          tunnel: [w1704] -> w1467 mode=indexing
          shift-right: [w1702] -> _
          shift-left: w1501 -> [w1712]
          tunnel: [w1697] -> w1461 mode=indexing
          tunnel: [w1696] -> w1460 mode=indexing
          tunnel: [w1695] -> w1459 mode=indexing
          tunnel: [w1694] -> w1458 mode=indexing
          tunnel: [w1685] -> w1457 mode=indexing
          tunnel: [w1684] -> w1455 mode=indexing
          tunnel: [w1683] -> w1454 mode=indexing
          tunnel: [w1682] -> w1453 mode=indexing
          tunnel: [w1681] -> w1452 mode=indexing
          tunnel: [w1680] -> w1451 mode=indexing
          tunnel: [w1679] -> w1450 mode=indexing
          tunnel: [w1678] -> w1449 mode=indexing
          tunnel: [w1660] -> w1431 mode=indexing
          i -> [w1703]
          n977 = Dequeue Element(queue=w1712) -> (queue out=w1702:refnum<queue>, element=w1661:dbl[][])  [unwired: 2 in, 2 out]
          n978 = Index Array(array=w1661, index (row)=29) -> ()  [unwired: 1 in, 1 out]
          n979 = Index Array(array=w1661, index (row)=27) -> ()  [unwired: 1 in, 1 out]
          n980 = Index Array(array=w1661, index (row)=28) -> ()  [unwired: 1 in, 1 out]
          n981 = Index Array(array=w1661, index (row)=25) -> ()  [unwired: 1 in, 1 out]
          n982 = Index Array(array=w1661, index (row)=26) -> ()  [unwired: 1 in, 1 out]
          n983 = Index Array(array=w1661, index (row)=24) -> ()  [unwired: 1 in, 1 out]
          n984 = Index Array(array=w1661, index (row)=30) -> ()  [unwired: 1 in, 1 out]
          n985 = Index Array(array=w1661, index (row)=31) -> ()  [unwired: 1 in, 1 out]
          n986 = Index Array(array=w1661, index (row)=23) -> ()  [unwired: 1 in, 1 out]
          n987 = Index Array(array=w1661, index (row)=22) -> ()  [unwired: 1 in, 1 out]
          n988 = Index Array(array=w1661, index (row)=20) -> ()  [unwired: 1 in, 1 out]
          n989 = Index Array(array=w1661, index (row)=13) -> (element=w1680:dbl[])  [unwired: 1 in]
          n990 = Index Array(array=w1661, index (row)=14) -> (element=w1679:dbl[])  [unwired: 1 in]
          n991 = Index Array(array=w1661, index (row)=15) -> (element=w1678:dbl[])  [unwired: 1 in]
          n992 = Index Array(array=w1661, index (row)=21) -> ()  [unwired: 1 in, 1 out]
          n993 = Index Array(array=w1661, index (row)=9) -> (element=w1684:dbl[])  [unwired: 1 in]
          n994 = Index Array(array=w1661, index (row)=10) -> (element=w1683:dbl[])  [unwired: 1 in]
          n995 = Index Array(array=w1661, index (row)=11) -> (element=w1682:dbl[])  [unwired: 1 in]
          n996 = Index Array(array=w1661, index (row)=12) -> (element=w1681:dbl[])  [unwired: 1 in]
          n997 = Index Array(array=w1661, index (row)=19) -> ()  [unwired: 1 in, 1 out]
          n998 = Index Array(array=w1661, index (row)=16) -> (element=w1660:dbl[])  [unwired: 1 in]
          n999 = Index Array(array=w1661, index (row)=18) -> ()  [unwired: 1 in, 1 out]
          n1000 = Index Array(array=w1661, index (row)=5) -> (element=w1696:dbl[])  [unwired: 1 in]
          n1001 = Index Array(array=w1661, index (row)=6) -> (element=w1695:dbl[])  [unwired: 1 in]
          n1002 = Index Array(array=w1661, index (row)=7) -> (element=w1694:dbl[])  [unwired: 1 in]
          n1003 = Index Array(array=w1661, index (row)=8) -> (element=w1685:dbl[])  [unwired: 1 in]
          n1004 = Index Array(array=w1661, index (row)=4) -> (element=w1697:dbl[])  [unwired: 1 in]
          n1005 = Index Array(array=w1661, index (row)=17) -> ()  [unwired: 1 in, 1 out]
          n1006 = Index Array(array=w1661, index (row)=1) -> (element=w1706:dbl[])  [unwired: 1 in]
          n1007 = Index Array(array=w1661, index (row)=2) -> (element=w1705:dbl[])  [unwired: 1 in]
          n1008 = Index Array(array=w1661, index (row)=3) -> (element=w1704:dbl[])  [unwired: 1 in]
          n1009 = Index Array(array=w1661, index (row)=0) -> (element=w1710:dbl[])  [unwired: 1 in]
          "NCS Save Loops" <- w1703
        }
        n1010 = for {
          N: w1435 -> [_]
          tunnel: [w1510] -> w1437 mode=concatenating
          tunnel: [w1507] -> w1438 mode=concatenating
          tunnel: [w1506] -> w1439 mode=concatenating
          tunnel: w1440 -> [w1503]
          tunnel: [w1502] -> w1436 mode=concatenating
          n1011 = Dequeue Element(queue=w1503) -> (element=w1504:dbl[][])  [unwired: 2 in, 3 out]
          n1012 = Index Array(array=w1504, index (row)=0) -> (element=w1506:dbl[])  [unwired: 1 in]
          n1013 = Index Array(array=w1504, index (row)=1) -> (element=w1507:dbl[])  [unwired: 1 in]
          n1014 = Index Array(array=w1504, index (row)=2) -> (element=w1510:dbl[])  [unwired: 1 in]
          n1015 = Index Array(array=w1504, index (row)=3) -> (element=w1502:dbl[])  [unwired: 1 in]
        }
        n1016 = local read "Current Routine"() -> (w1498:string)
        n1017 = local read "Case #"() -> (w1434:string)
        n1018 = Concatenate Strings("Case", w1434, w1498) -> (w1432:string)
        n1019 = flat-sequence {
          tunnel: w1474 -> [w1594]
          tunnel: w1475 -> [w1595]
          tunnel: w1476 -> [w1596]
          tunnel: w1477 -> [w1597]
          tunnel: w1478 -> [w1599]
          tunnel: w1479 -> [w1598]
          tunnel: w1480 -> [w1600]
          tunnel: w1481 -> [w1601]
          tunnel: w1482 -> [w1602]
          tunnel: w1483 -> [w1603]
          tunnel: w1484 -> [w1604]
          tunnel: w1485 -> [w1605]
          tunnel: w1486 -> [w1606]
          tunnel: w1487 -> [w1607]
          tunnel: "Abd (cm)" -> [w1629]
          tunnel: "Comments" -> [w1624]
          tunnel: "Weight (lbs)" -> [w1625]
          tunnel: "Thorax (cm)" -> [w1627]
          tunnel: "Height (cm)" -> [w1632]
          tunnel: "Age (yrs)" -> [w1634]
          tunnel: "Sex" -> [w1636]
          tunnel: "Case #" -> [w1637]
          tunnel: path "C:/Users/Edwin Kan Group/Documents/Zijing/dyspnea stuC:/Users/Edwin Kan Group/Documents/Zijing/dyspnea study/data/10_12" ("base path") -> [w1658]
          tunnel: w1432 -> [w1657]
          tunnel: w1473 -> [w1593]
          tunnel: w1466 -> [w1580]
          tunnel: w1468 -> [w1583]
          tunnel: w1470 -> [w1588]
          tunnel: w1465 -> [w1579]
          tunnel: w1464 -> [w1576]
          tunnel: w1463 -> [w1571]
          tunnel: w1462 -> [w1570]
          tunnel: w1448 -> [w1565]
          tunnel: w1447 -> [w1562]
          tunnel: w1446 -> [w1559]
          tunnel: w1445 -> [w1556]
          tunnel: w1444 -> [w1555]
          tunnel: w1443 -> [w1548]
          tunnel: w1442 -> [w1547]
          tunnel: w1441 -> [w1546]
          tunnel: w1439 -> [w1519]
          tunnel: w1438 -> [w1517]
          tunnel: w1437 -> [w1515]
          tunnel: w1436 -> [w1513]
          frame #0 {
            n1020 = Build Path(base path=w1658, name or relative path=w1657) -> (appended path=w1640:path)
            n1021 = TDMS Open(6:FALSE ("disable buffering (T)"), 10:T9."open or create" ("operation"), 11:w1640) -> (0:w1655:errorcluster, 3:w1656:refnum<k34>)  [unwired: 4 in]
            n1022 = TDMS Set Properties(5:w1637, 7:"Case Number", 8:w1655, 11:w1656) -> (0:w1654:errorcluster, 3:w1653:refnum<k34>)  [unwired: 2 in, 2 out]
            n1023 = TDMS Set Properties(5:w1636, 7:"Sex", 8:w1654, 11:w1653) -> (0:w1652:errorcluster, 3:w1651:refnum<k34>)  [unwired: 2 in, 2 out]
            n1024 = TDMS Set Properties(5:w1634, 7:"Age (years)", 8:w1652, 11:w1651) -> (0:w1650:errorcluster, 3:w1649:refnum<k34>)  [unwired: 2 in, 2 out]
            n1025 = TDMS Set Properties(5:w1632, 7:"Height (cm)", 8:w1650, 11:w1649) -> (0:w1647:errorcluster, 3:w1646:refnum<k34>)  [unwired: 2 in, 2 out]
            n1026 = TDMS Set Properties(5:w1629, 7:"AbdCircumference (cm)", 8:w1647, 11:w1646) -> (0:w1645:errorcluster, 3:w1644:refnum<k34>)  [unwired: 2 in, 2 out]
            n1027 = TDMS Set Properties(5:w1627, 7:"Thorax Circumference (cm)", 8:w1645, 11:w1644) -> (0:w1642:errorcluster, 3:w1643:refnum<k34>)  [unwired: 2 in, 2 out]
            n1028 = TDMS Set Properties(5:w1625, 7:"Weight (lbs)", 8:w1642, 11:w1643) -> (0:w1626:errorcluster, 3:w1648:refnum<k34>)  [unwired: 2 in, 2 out]
            n1029 = TDMS Set Properties(5:w1624, 7:"Comments", 8:w1626, 11:w1648) -> (0:w1608:errorcluster, 3:w1609:refnum<k34>)  [unwired: 2 in, 2 out]
            n1030 = TDMS Set Properties(5:w1606, 7:w1607, 8:w1608, 11:w1609) -> (0:w1621:errorcluster, 3:w1620:refnum<k34>)  [unwired: 2 in, 2 out]
            n1031 = TDMS Set Properties(5:w1604, 7:w1605, 8:w1621, 11:w1620) -> (0:w1619:errorcluster, 3:w1618:refnum<k34>)  [unwired: 2 in, 2 out]
            n1032 = TDMS Set Properties(5:w1602, 7:w1603, 8:w1619, 11:w1618) -> (0:w1616:errorcluster, 3:w1615:refnum<k34>)  [unwired: 2 in, 2 out]
            n1033 = TDMS Set Properties(5:w1600, 7:w1601, 8:w1616, 11:w1615) -> (0:w1614:errorcluster, 3:w1613:refnum<k34>)  [unwired: 2 in, 2 out]
            n1034 = TDMS Set Properties(5:w1598, 7:w1599, 8:w1614, 11:w1613) -> (0:w1611:errorcluster, 3:w1612:refnum<k34>)  [unwired: 2 in, 2 out]
            n1035 = TDMS Set Properties(5:w1596, 7:w1597, 8:w1611, 11:w1612) -> (0:w1610:errorcluster, 3:w1617:refnum<k34>)  [unwired: 2 in, 2 out]
            n1036 = TDMS Set Properties(5:w1594, 7:w1595, 8:w1610, 11:w1617) -> (0:w1591:errorcluster, 3:w1592:refnum<k34>)  [unwired: 2 in, 2 out]
            n1037 = TDMS Write(0:w1592, 7:"Tx1Rx1", 9:w1593, 11:w1591) -> (4:w1589:refnum<k34>, 15:w1590:errorcluster)  [unwired: 2 in, 2 out]
            n1038 = TDMS Write(0:w1589, 7:"Tx2Rx1", 9:w1588, 11:w1590) -> (4:w1584:refnum<k34>, 15:w1585:errorcluster)  [unwired: 2 in, 2 out]
            n1039 = TDMS Write(0:w1584, 7:"Tx3Rx1", 9:w1583, 11:w1585) -> (4:w1581:refnum<k34>, 15:w1582:errorcluster)  [unwired: 2 in, 2 out]
            n1040 = TDMS Write(0:w1581, 7:"Tx4Rx1", 9:w1580, 11:w1582) -> (4:w1577:refnum<k34>, 15:w1578:errorcluster)  [unwired: 2 in, 2 out]
            n1041 = TDMS Write(0:w1577, 7:"Tx1Rx2", 9:w1579, 11:w1578) -> (4:w1574:refnum<k34>, 15:w1575:errorcluster)  [unwired: 2 in, 2 out]
            n1042 = TDMS Write(0:w1574, 7:"Tx2Rx2", 9:w1576, 11:w1575) -> (4:w1572:refnum<k34>, 15:w1573:errorcluster)  [unwired: 2 in, 2 out]
            n1043 = TDMS Write(0:w1572, 7:"Tx3Rx2", 9:w1571, 11:w1573) -> (4:w1568:refnum<k34>, 15:w1569:errorcluster)  [unwired: 2 in, 2 out]
            n1044 = TDMS Write(0:w1568, 7:"Tx4Rx2", 9:w1570, 11:w1569) -> (4:w1566:refnum<k34>, 15:w1567:errorcluster)  [unwired: 2 in, 2 out]
            n1045 = TDMS Write(0:w1566, 7:"Tx1Rx3", 9:w1565, 11:w1567) -> (4:w1563:refnum<k34>, 15:w1564:errorcluster)  [unwired: 2 in, 2 out]
            n1046 = TDMS Write(0:w1563, 7:"Tx2Rx3", 9:w1562, 11:w1564) -> (4:w1561:refnum<k34>, 15:w1558:errorcluster)  [unwired: 2 in, 2 out]
            n1047 = TDMS Write(0:w1561, 7:"Tx3Rx3", 9:w1559, 11:w1558) -> (4:w1560:refnum<k34>, 15:w1557:errorcluster)  [unwired: 2 in, 2 out]
            n1048 = TDMS Write(0:w1560, 7:"Tx4Rx3", 9:w1556, 11:w1557) -> (4:w1553:refnum<k34>, 15:w1554:errorcluster)  [unwired: 2 in, 2 out]
            n1049 = TDMS Write(0:w1553, 7:"Tx1Rx4", 9:w1555, 11:w1554) -> (4:w1552:refnum<k34>, 15:w1551:errorcluster)  [unwired: 2 in, 2 out]
            n1050 = TDMS Write(0:w1552, 7:"Tx2Rx4", 9:w1548, 11:w1551) -> (4:w1549:refnum<k34>, 15:w1550:errorcluster)  [unwired: 2 in, 2 out]
            n1051 = TDMS Write(0:w1549, 7:"Tx3Rx4", 9:w1547, 11:w1550) -> (4:w1544:refnum<k34>, 15:w1545:errorcluster)  [unwired: 2 in, 2 out]
            n1052 = TDMS Write(0:w1544, 7:"Tx4Rx4", 9:w1546, 11:w1545) -> (4:w1529:refnum<k34>, 15:w1524:errorcluster)  [unwired: 2 in, 2 out]
            n1053 = TDMS Write(0:w1529, 7:"BIOPAC_CH1", 9:w1519, 11:w1524) -> (4:w1528:refnum<k34>, 15:w1523:errorcluster)  [unwired: 2 in, 2 out]
            n1054 = TDMS Write(0:w1528, 7:"BIOPAC_CH2", 9:w1517, 11:w1523) -> (4:w1527:refnum<k34>, 15:w1522:errorcluster)  [unwired: 2 in, 2 out]
            n1055 = TDMS Write(0:w1527, 7:"BIOPAC_CH3", 9:w1515, 11:w1522) -> (4:w1526:refnum<k34>, 15:w1521:errorcluster)  [unwired: 2 in, 2 out]
            n1056 = TDMS Write(0:w1526, 7:"BIOPAC_CH4", 9:w1513, 11:w1521) -> (4:w1525:refnum<k34>, 15:w1520:errorcluster)  [unwired: 2 in, 2 out]
            n1057 = TDMS Close(8:w1520, 11:w1525) -> ()  [unwired: 2 out]
          }
          frame #1 {
            n1058 = local write "Save"(FALSE) -> ()
          }
        }
        n1059 = local read "Start Time"() -> (w1490:T2)
        n1060 = property on="fractional second" class="DigNum (strict)"() -> ("Label.Text"=w1487:string)  [unwired: 2 in, 2 out]
        n1061 = property on="second" class="DigNum (strict)"() -> ("Label.Text"=w1485:string)  [unwired: 2 in, 2 out]
        n1062 = Unbundle By Name(w1490) -> ("fractional second"=w1486:dbl, "second"=w1484:i32, "minute"=w1482:i32, "hour"=w1480:i32, "day of month"=w1479:i32, "month"=w1476:i32, "year"=w1474:i32)
        n1063 = property on="minute" class="DigNum (strict)"() -> ("Label.Text"=w1483:string)  [unwired: 2 in, 2 out]
        n1064 = property on="hour" class="DigNum (strict)"() -> ("Label.Text"=w1481:string)  [unwired: 2 in, 2 out]
        n1065 = property on="month" class="DigNum (strict)"() -> ("Label.Text"=w1477:string)  [unwired: 2 in, 2 out]
        n1066 = property on="day of month" class="DigNum (strict)"() -> ("Label.Text"=w1478:string)  [unwired: 2 in, 2 out]
        n1067 = property on="year" class="DigNum (strict)"() -> ("Label.Text"=w1475:string)  [unwired: 2 in, 2 out]
        n1068 = Reshape Array(w1472, w1456) -> (w1473:dbl[])
        n1069 = Reshape Array(w1471, w1456) -> (w1470:dbl[])
        n1070 = Reshape Array(w1469, w1456) -> (w1468:dbl[])
        n1071 = Reshape Array(w1467, w1456) -> (w1466:dbl[])
        n1072 = Reshape Array(w1461, w1456) -> (w1465:dbl[])
        n1073 = Reshape Array(w1460, w1456) -> (w1464:dbl[])
        n1074 = Reshape Array(w1459, w1456) -> (w1463:dbl[])
        n1075 = Reshape Array(w1458, w1456) -> (w1462:dbl[])
        n1076 = Reshape Array(w1457, w1456) -> (w1448:dbl[])
        n1077 = Reshape Array(w1455, w1456) -> (w1447:dbl[])
        n1078 = Reshape Array(w1454, w1456) -> (w1446:dbl[])
        n1079 = Reshape Array(w1453, w1456) -> (w1445:dbl[])
        n1080 = Reshape Array(w1452, w1456) -> (w1444:dbl[])
        n1081 = Reshape Array(w1451, w1456) -> (w1443:dbl[])
        n1082 = Reshape Array(w1450, w1456) -> (w1442:dbl[])
        n1083 = Reshape Array(w1449, w1456) -> (w1441:dbl[])
      }
    }
  }
  n1084 = while {
    stop <- FALSE stop-if-true
    # "Viewing NCS"
    n1085 = local read "8 Ch Heart"() -> (w1720:dbl[][])
    n1086 = Index Array(array=w1720, index (row)=6 ("index")) -> (element=w1718:dbl[])  [unwired: 1 in]
    n1087 = Index Array(array=w1720, index (row)=7 ("index")) -> (element=→"Tx3Rx4":dbl[])  [unwired: 1 in]
    n1088 = Index Array(array=w1720, index (row)=3 ("index")) -> (element=→"Tx1Rx2":dbl[])  [unwired: 1 in]
    n1089 = Index Array(array=w1720, index (row)=2 ("index")) -> (element=w1723:dbl[])  [unwired: 1 in]
    n1090 = Index Array(array=w1720, index (row)=0 ("index")) -> (element=w1725:dbl[])  [unwired: 1 in]
    n1091 = Index Array(array=w1720, index (row)=5 ("index")) -> (element=→"Tx4Rx3":dbl[])  [unwired: 1 in]
    n1092 = Index Array(array=w1720, index (row)=4 ("index")) -> (element=w1721:dbl[])  [unwired: 1 in]
    n1093 = Index Array(array=w1720, index (row)=1 ("index")) -> (element=→"Tx2Rx1":dbl[])  [unwired: 1 in]
    n1094 = Wait (ms)(milliseconds to wait=u32 30) -> ()  [unwired: 1 out]
  }
  "error out 1" <- w169
  "error out 2" <- w103
  "DownSamplingRatio" <- "DownSamplingRatio1"
  "ACQ ms" <- 100.0
  "Connecting" <- w1
  "Stopping" <- w1
  "Disconnecting" <- w1
  "Boolean" <- TRUE
  "Disconnected" <- w1
  "Connected" <- w1
  "Receive Success" <- w1
  "Receiving" <- w1
  "Acq Started" <- w1
